vi "AMC100 UI.vi"() -> ()   [LabVIEW 2016]
panel:
  in  "stop":bool
  in  "Tab Control":enum32{"Navigation", "Interface", "About"}(tab)
  out "move out":bool caption="Move"
  in  "Positioner 2":u16(ring)=15 caption="Positioner" items=["ECGp5050", "ECGt5050", "ECR3030", "ECR4040", "ECR5050", "ECSx3030", "ECSx3040", "ECSx3050", "ECSx3060", "ECSx3070", "ECSx3080", "ECSx5050", "ECSxy5050", "ECSz3030", "ECSz5050", "EOP1", "EOP2"]
  out "in target range3":bool
  in  "Target Range 3":u32 caption="Target Range"
  in  "Reset Error 2":bool
  in  "Reset Error 3":bool
  out "Error 3":bool caption="Error"
  out "Error Message 3":string
  out "actor type 3":u16(ring) caption="Status" items=["linear positioner"=0, "goniometer"=1, "rotator"=2, "< error >"=9]
  out "actor type 2":u16(ring) caption="Status" items=["linear positioner"=0, "rotator"=1, "goniometer"=2, "< error >"=9]
  out "actor type":u16(ring) caption="Status" items=["linear positioner"=0, "rotator"=1, "goniometer"=2, "< error >"=9]
  out "EotLeftDetected3":bool caption="Status Eot BWD"
  out "EotrightDetected3":bool caption="Status Eot FWD"
  in  "EoT 3":bool=TRUE caption="Stop on EoT"
  out "EotLeftDetected2":bool caption="Status Eot BWD"
  out "EotrightDetected2":bool caption="Status Eot FWD"
  in  "EoT 2":bool=TRUE caption="Stop on EoT"
  in  "Move 3":bool
  out "MoveSignal 3":bool caption="Move"
  out "MoveSignal":bool caption="Move"
  out "ReferenceSignal":bool=TRUE
  in  "Axis 3":bool caption="Closed Loop Funktions"
  in  "Axis 2":bool caption="Closed Loop Funktions"
  in  "Target Position 3":i32 caption="Target Position [µm]"
  in  "Target Position 1":i32 caption="Target position [µm]"
  in  "Number of steps 3":i32=1 caption="Number of Steps"
  in  "Number of steps 2":i32=1 caption="Number of Steps"
  in  "Output 2":bool caption="Axis 2"
  in  "Move 2":bool
  in  "Move":bool
  out "ReferenceSignal 3":bool
  out "Reference 3":dbl caption="Reference position [µm]" format="%#_6f"
  in  "Output":bool=TRUE caption="Axis 1"
  out "Output Status 3":bool caption="Output Status"
  out "Error Message":string
  out "Error":bool
  in  "Output 3":bool caption="Axis 3"
  out "Output Status 1":bool=TRUE caption="Output Status"
  out "Position 3":dbl caption="Position [µm]" format="%#_10g"
  out "Output Status 2":bool caption="Output Status"
  in  "auto Reset 3":bool=TRUE caption="Auto Reset"
  in  "amplitude [V] 3":dbl=45.001 caption="Amplitude [V]" format="%#.3f"
  in  "frequency [Hz] 3":dbl=997.363 caption="Frequency [Hz]" format="%#.3f"
  out "Error 2":bool caption="Error"
  out "Error Message 2":string
  out "Connected 3":bool caption="Positioner Connected/Moving"
  in  "Single Step Left 3":bool caption="Open Loop Funktions"
  in  "Positioner 3":u16(ring)=15 caption="Positioner" items=["ECGp5050", "ECGt5050", "ECR3030", "ECR4040", "ECR5050", "ECSx3030", "ECSx3040", "ECSx3050", "ECSx3060", "ECSx3070", "ECSx3080", "ECSx5050", "ECSxy5050", "ECSz3030", "ECSz5050", "EOP1", "EOP2"]
  in  "Endless Left 3":bool caption="Continuous Backward"
  in  "Continuous Forward":bool
  in  "Single Step Right 3":bool caption="Step(s)"
  in  "Fixed DC 3":i32 caption="DC Level"
  out "move out 3":bool caption="Move"
  out "Position 2":i32 caption="Position [µm]"
  in  "amplitude [V] 2":dbl=45.001 caption="Amplitude [V]" format="%#.3f"
  in  "Reference Auto Update 3":bool=TRUE caption="Auto Update"
  in  "Amplitude [V]":dbl=45.001 format="%#.3f"
  in  "frequency [Hz] 2":dbl=997.363 caption="Frequency [Hz]" format="%#.3f"
  in  "Reference Auto Update 1":bool=TRUE caption="Auto Update"
  in  "Frequency [Hz]":dbl=1998.531 format="%#.3f"
  out "Connected 2":bool caption="Positioner Connected/Moving"
  in  "Single Step Left":bool caption="Open Loop Funktions"
  in  "Single Step Left 2":bool caption="Open Loop Funktions"
  in  "Single Step Right 2":bool caption="Step(s)"
  in  "Number of steps 1":i32=1 caption="Number of Steps"
  out "ReferenceSignal 2":bool
  in  "Single Step Right":bool caption="Step(s)"
  in  "Endless Left":bool caption="Continuous Backward"
  in  "Continuous Forward":bool
  in  "Endless Left 2":bool caption="Continuous Backward"
  out "EotLeftDetected1":bool caption="Status Eot BWD"
  out "EotrightDetected1":bool caption="Status Eot FWD"
  in  "EoT 1":bool caption="Stop on EoT"
  in  "Target position 2":i32 caption="Target Position [µm]"
  out "in target range2":bool
  in  "Continuous Forward":bool
  out "Reference 2":i32 caption="Reference position [µm]"
  in  "Fixed DC 2":i32 caption="DC Level"
  out "MoveSignal 2":bool caption="Move"
  out "in target range1":bool
  in  "Target Range 2":u32 caption="Target Range"
  in  "Target Range 1":u32 caption="Target Range"
  out "Reference":dbl=-7597148.0 caption="Reference position [µm]" format="%#_6f"
  out "Position":dbl=14701.126 caption="Position [µm]" format="%#_10f"
  in  "Axis 1":bool caption="Closed Loop Funktions"
  in  "auto Reset 1":bool=TRUE caption="Auto Reset"
  in  "Fixed DC 1":i32 caption="DC Level"
  out "move out 2":bool caption="Move"
  in  "auto Reset 2":bool=TRUE caption="Auto Reset"
  in  "Reference Auto Update 2":bool=TRUE caption="Auto Update"
  in  "Reset Error":bool
  out "Connected":bool=TRUE caption="Positioner Connected/Moving"
  in  "Positioner":u16(ring)=15 items=["ECGp5050", "ECGt5050", "ECR3030", "ECR4040", "ECR5050", "ECSx3030", "ECSx3040", "ECSx3050", "ECSx3060", "ECSx3070", "ECSx3080", "ECSx5050", "ECSxy5050", "ECSz3030", "ECSz5050", "EOP1", "EOP2"]
  in  "RT in move 3":bool=TRUE caption="Move"
  in  "Steps per pulse 3":i32 caption="Steps per pulse [Steps]"
  out "RT in move Signal 3":bool=TRUE caption="move"
  in  "Mode Input 3":u16(ring) caption="Mode" items=["Trigger (LVDS)"=11, "Trigger (LVTTL)"=10, "Stepper (LVDS)"=9, "Stepper (LVTTL)"=8, "AquadB (LVDS)"=1, "AquadB (LVTTL)"=0, "OFF"=15]
  in  "Loop Mode 3":u16(ring) caption="Loop mode" items=["closed-loop"=1, "open-loop"=0]
  in  "Change per pulse 3":i32 caption="Change per pulse  [u°/nm]"
  in  "RT in move 2":bool=TRUE caption="Move"
  in  "Steps per pulse 2":i32 caption="Steps per pulse [Steps]"
  out "RT in move Signal 2":bool=TRUE caption="move"
  in  "Mode Input 2":u16(ring) caption="Mode" items=["Trigger (LVDS)"=11, "Trigger (LVTTL)"=10, "Stepper (LVDS)"=9, "Stepper (LVTTL)"=8, "AquadB (LVDS)"=1, "AquadB (LVTTL)"=0, "OFF"=15]
  in  "Loop Mode 2":u16(ring) caption="Loop mode" items=["closed-loop"=1, "open-loop"=0]
  in  "Change per pulse 2":i32 caption="Change per pulse  [u°/nm]"
  in  "Output Mode":u16(ring) caption="Mode" items=["AquadB (LVTTL)", "AquadB (LVDS)"]
  in  "RT in move 1":bool=TRUE caption="Move"
  in  "AquadB Resolution 3":i32 caption="AquadB Resolution [nm]"
  in  "AqaudB clock 2":i32 caption="AquadB Clock [ns]"
  in  "AqaudB clock 1":i32 caption="AquadB Clock [ns]"
  in  "AquadB Resolution 2":i32 caption="AquadB Resolution [nm]"
  in  "AquadB out 1":bool caption="AquadB enable"
  in  "Steps per pulse 1":i32 caption="Steps per pulse [Steps]"
  in  "AquadB out 3":bool caption="AquadB enable"
  in  "AquadB in res 1":i32 caption="AquadB Resolution [nm]"
  in  "AquadB Resolution 1":i32 caption="AquadB Resolution [nm]"
  in  "AquadB out 2":bool caption="AquadB enable"
  in  "AqaudB clock 3":i32 caption="AquadB Clock [ns]"
  in  "Reset Error 6":bool
  in  "Reset Error 5":bool
  out "Error Message 5":string
  out "Error 5":bool caption="Error"
  out "Error Message 6":string
  out "Error 6":bool caption="Error"
  in  "AquadB in res 3":i32 caption="AquadB Resolution [nm]"
  in  "AquadB in res 2":i32 caption="AquadB Resolution [nm]"
  in  "Reset Error 4":bool
  out "RT in move Signal 1":bool=TRUE caption="move"
  in  "Mode Input 1":u16(ring) caption="Mode" items=["Trigger (LVDS)"=11, "Trigger (LVTTL)"=10, "Stepper (LVDS)"=9, "Stepper (LVTTL)"=8, "AquadB (LVDS)"=1, "AquadB (LVTTL)"=0, "OFF"=15]
  out "Error Message 4":string
  out "Error 4":bool caption="Error"
  in  "Loop Mode 1":u16(ring) caption="Loop mode" items=["closed-loop"=1, "open-loop"=0]
  in  "Change per pulse 1":i32 caption="Change per pulse [u°/nm]"
  in  "Reset Error 7":bool
  in  "Factory Reset":bool
  in  "Reboot":bool
  out "Error Message 7":string
  in  "Lock password":string
  in  "name":string caption="Device Name"
  in  "Access Password":string
  out "locked":bool
  out "authorized":bool
  out "Error 7":bool caption="Error"
  in  "Unlock":bool=TRUE
  out "Name":string caption="Device Name"
  out "Device type":string="AMC100/NUM"
  out "Mac Adress":string="70:B3:D5:D7:61:E1"
  out "Sn":string caption="Serial Number"
  out "ip":string="192.168.1.1" caption="IP Adress"
  out "Firmware":string caption="Firmware Version"
  out "FPGA":string caption="FPGA Version"
  # "Real Time Output"
  # "Real Time Input"
  # "Global Parameters"
  # "Axis 1"
  # "Axis 1"
  # "Axis 2"
  # "Axis 2"
  # "Axis 3"
  # "Axis 3"
  # "Device Info"
  # "Device Access"
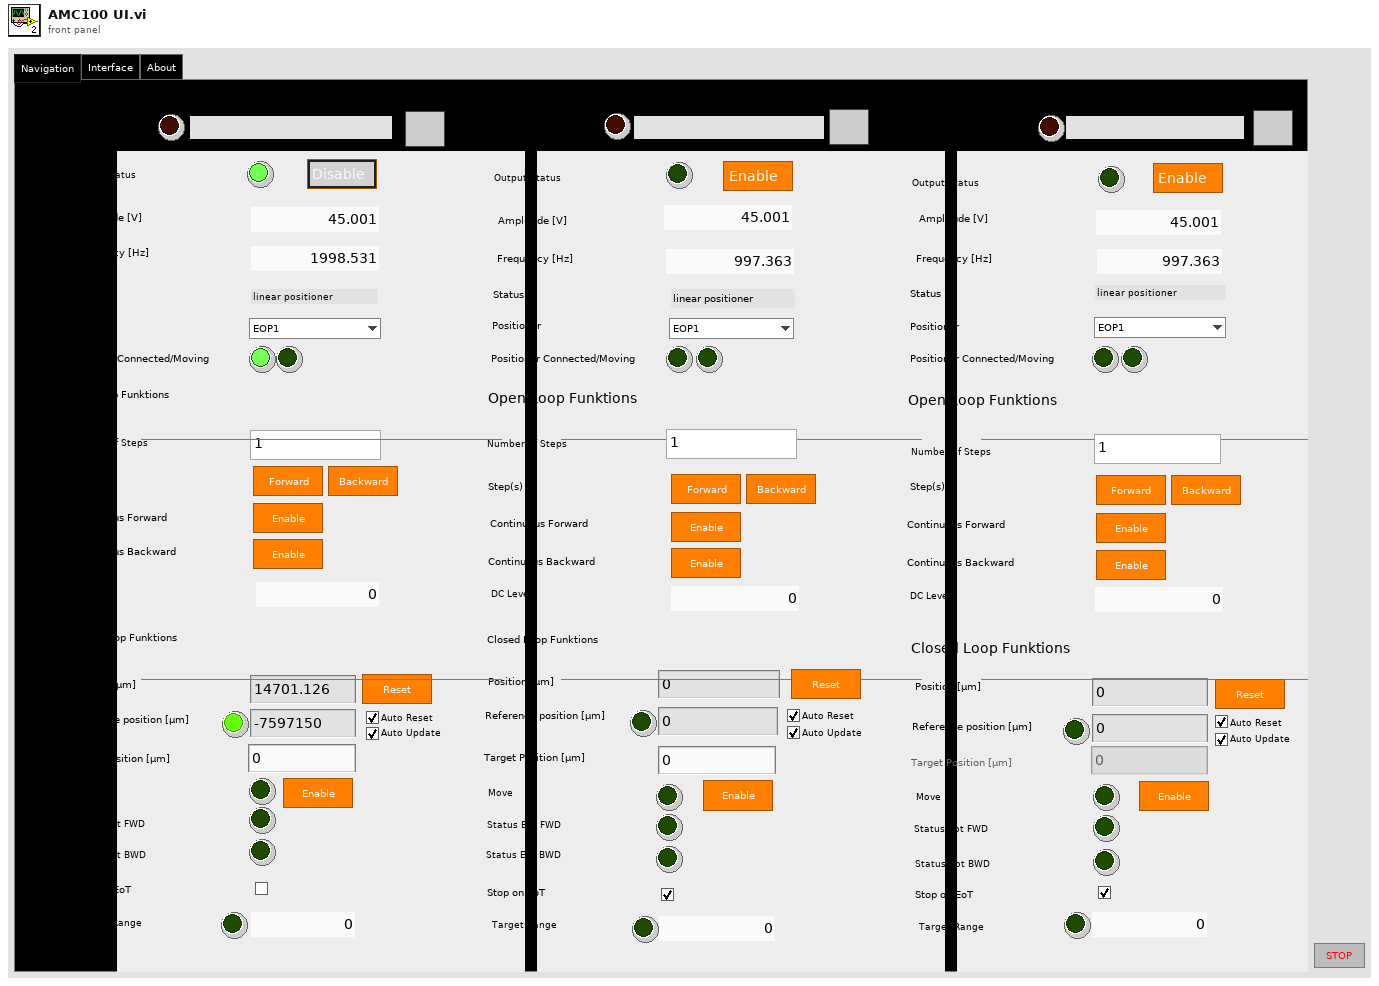
[diagram p1: front panel]
types:
  T1 = enum8{"Enabled", "Disabled", "Disabled and Grayed Out"}
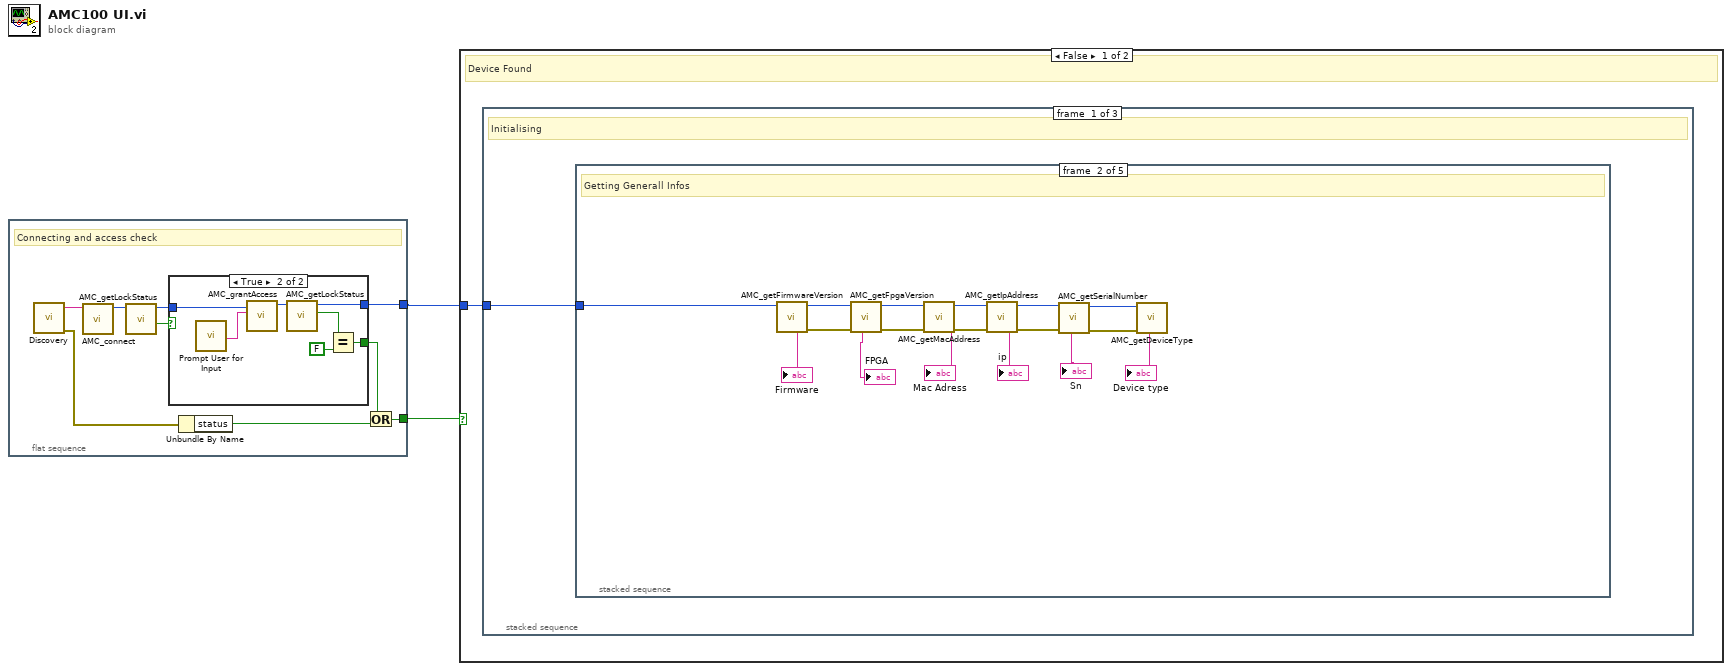
[diagram p0: block diagram]
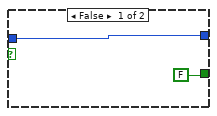
[diagram p2: hidden frame]
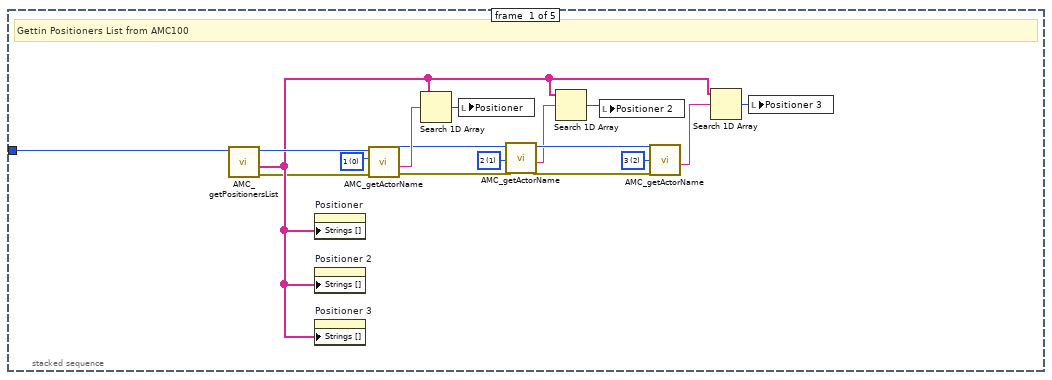
[diagram p3: hidden frame]
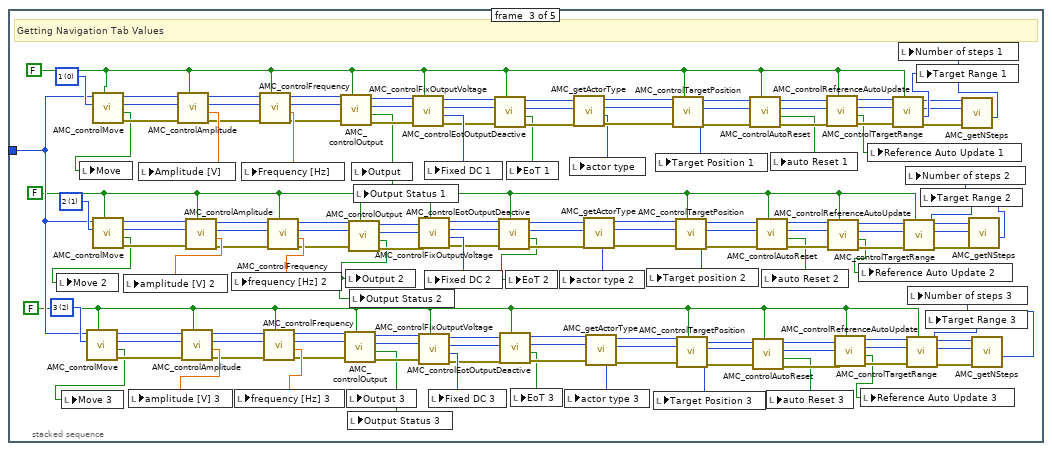
[diagram p4: hidden frame]
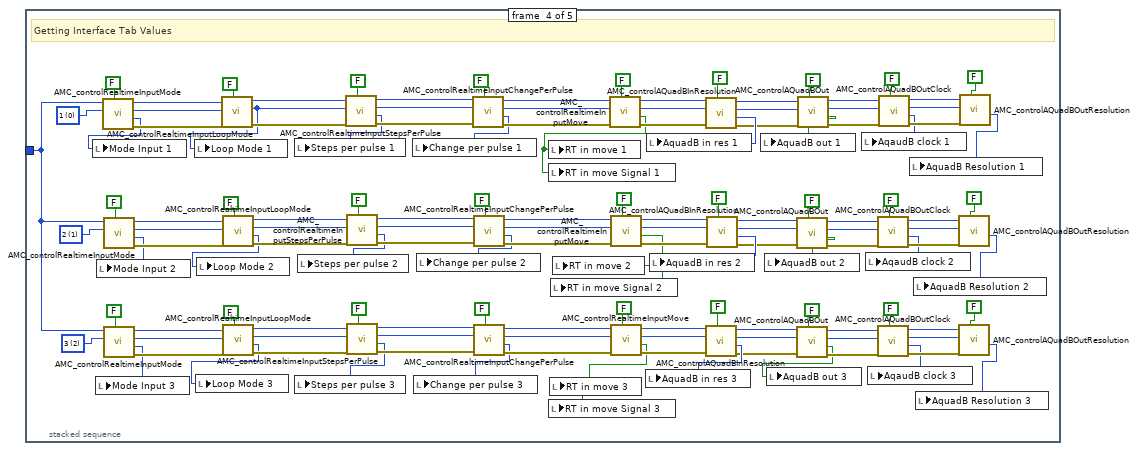
[diagram p5: hidden frame]
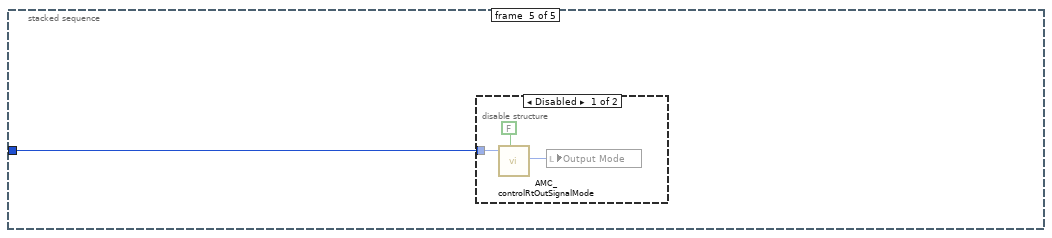
[diagram p6: hidden frame]
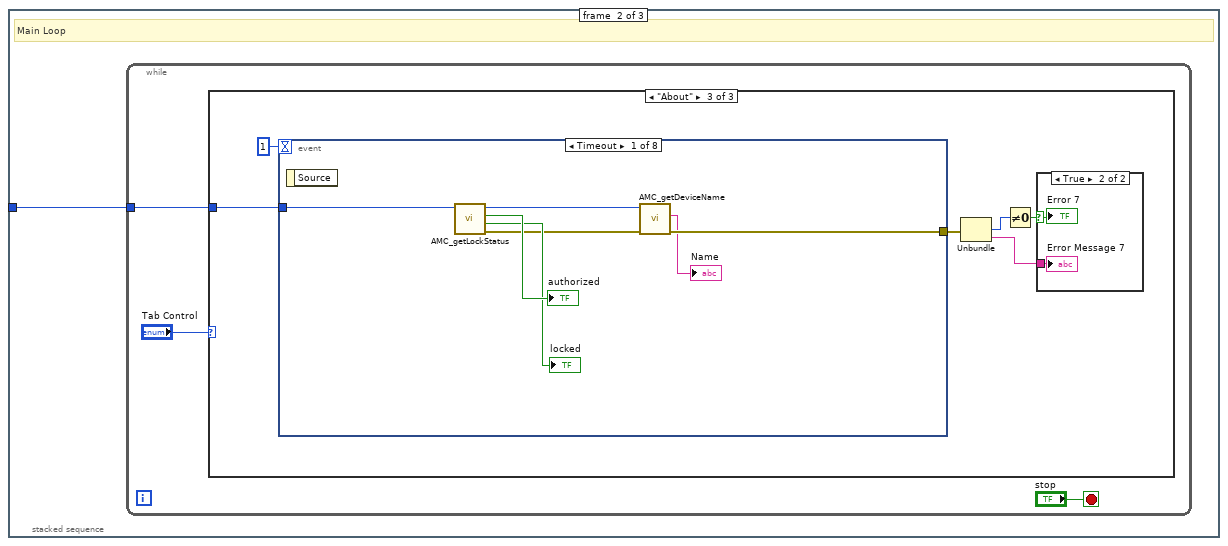
[diagram p8: hidden frame]
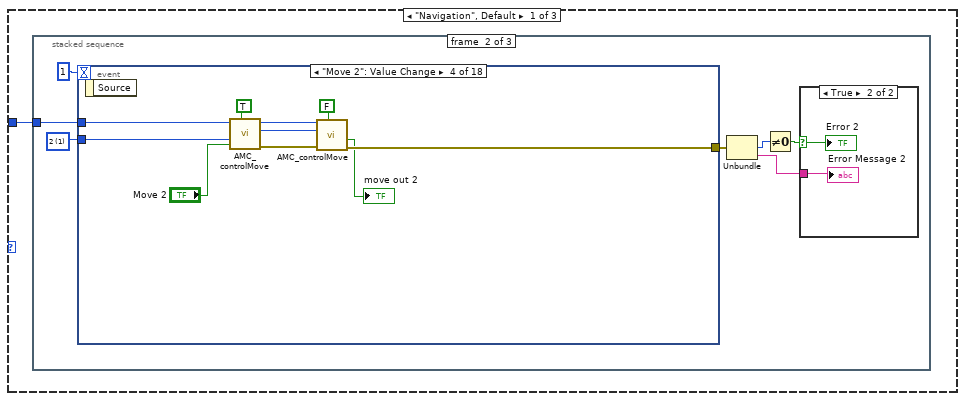
[diagram p9: hidden frame]
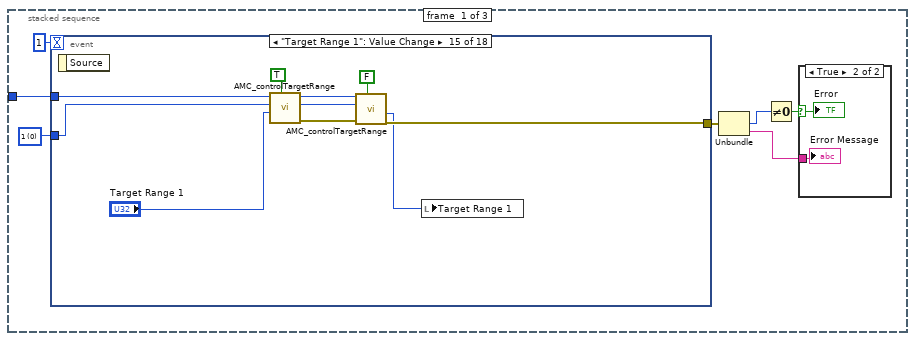
[diagram p10: hidden frame]
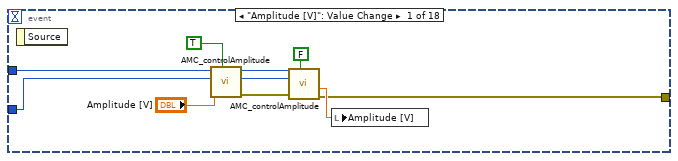
[diagram p12: hidden frame]
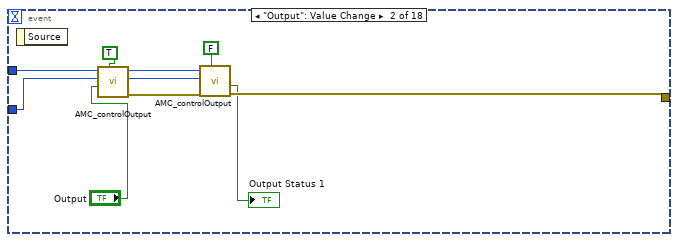
[diagram p13: hidden frame]
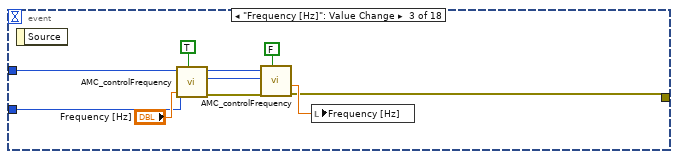
[diagram p14: hidden frame]
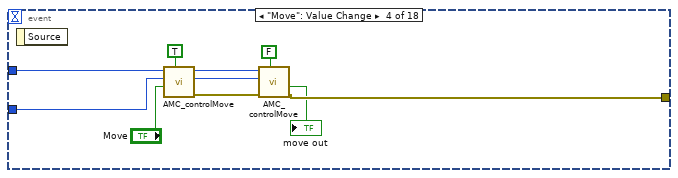
[diagram p15: hidden frame]
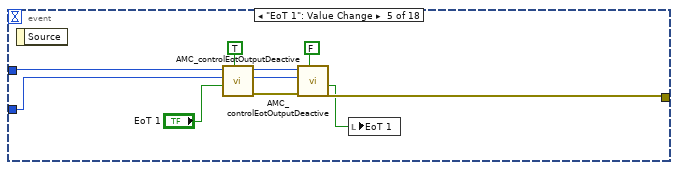
[diagram p16: hidden frame]
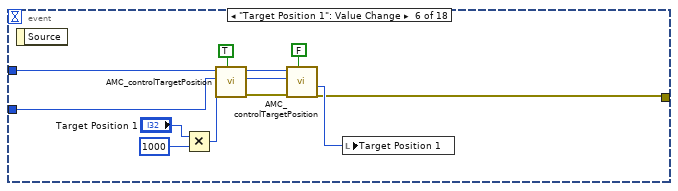
[diagram p17: hidden frame]
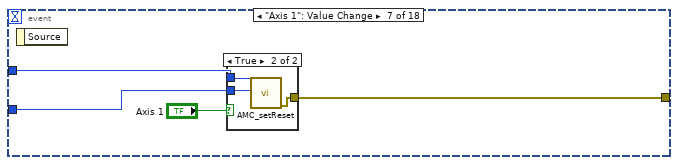
[diagram p18: hidden frame]
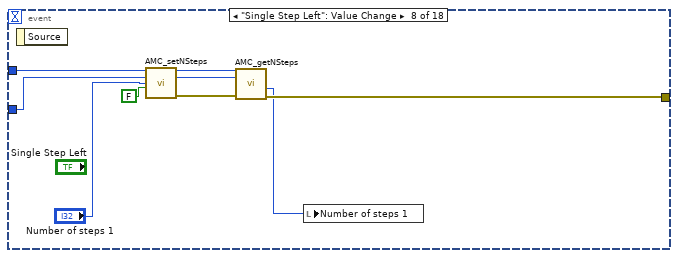
[diagram p20: hidden frame]
diagram:
  n1 = flat-sequence {
    tunnel: [w10] -> w1
    tunnel: [w11] -> w2
    frame #0 {
      # "Connecting and access check"
      n2 = call "Discovery.vi"() -> ("error out"=w3:errorcluster, "IP"=w4:string)  [unwired: 10 in]
      n3 = call "AMC_connect.vi"("deviceAddress"=w4) -> ("deviceHandle"=w7:i32)  [unwired: 5 in, 1 out]
      n4 = call "AMC_getLockStatus.vi"("deviceHandle"=w7) -> ("locked"=w5:bool, "deviceHandle"=w6:i32)  [unwired: 7 in, 2 out]
      n5 = case shown="True" w5 {
        tunnel: w6 -> [w13 w20]
        tunnel: [w13 w17] -> w11
        tunnel: [FALSE w14] -> w9
        frame False {
        }
        frame True {
          n6 = call "Prompt User for Input"() -> ("password"=w19:string)  [unwired: 17 in, 2 out]
          n7 = call "AMC_grantAccess.vi"("password"=w19, "deviceHandle"=w20) -> ("deviceHandle"=w18:i32)  [unwired: 8 in, 1 out]
          n8 = call "AMC_getLockStatus.vi"("deviceHandle"=w18) -> ("authorized"=w15:bool, "deviceHandle"=w17:i32)  [unwired: 7 in, 2 out]
          n9 = Equal?(x=w15, y=FALSE) -> (x = y?=w14:bool)
        }
      }
      n10 = Unbundle By Name(w3) -> ("status"=w8:bool)
      n11 = Or(x=w9, y=w8) -> (x .or. y?=w10:bool)
    }
  }
  n12 = case shown="False" w1 {
    tunnel: w2 -> [w21 _]
    frame False {
      # "Device Found"
      n13 = stacked-sequence {
        tunnel: w21 -> [w22 w332 w1333]
        frame #0 {
          # "Initialising"
          n14 = stacked-sequence {
            tunnel: w22 -> [w32 w44 w102 w278 w328]
            frame #0 {
              w34 = u8 2 items=["1", "2", "3"] ("axis")
              w33 = u8 1 items=["1", "2", "3"] ("axis")
              w37 = u8 0 items=["1", "2", "3"] ("axis")
              # "Gettin Positioners List from AMC100"
              n15 = call "AMC_getPositionersList.vi"("deviceHandle"=w32) -> ("error out"=w23:errorcluster, "list"=w26:string[], "deviceHandle"=w27:i32)  [unwired: 7 in, 1 out]
              n16 = property on="Positioner" class="Ring (strict)"("Strings []"=w26) -> ()  [unwired: 2 in, 2 out]
              n17 = property on="Positioner 2" class="Ring (strict)"("Strings []"=w26) -> ()  [unwired: 2 in, 2 out]
              n18 = property on="Positioner 3" class="Ring (strict)"("Strings []"=w26) -> ()  [unwired: 2 in, 2 out]
              n19 = call "AMC_getActorName.vi"("error in"=w23, "axis"=w37, "deviceHandle"=w27) -> ("error out"=w25:errorcluster, "actor name"=w38:string, "deviceHandle"=w36:i32)  [unwired: 5 in, 1 out]
              n20 = Search 1D Array(1D array=w26, element=w38) -> (index of element=w39:i32)  [unwired: 1 in]
              n21 = local write "Positioner"(w39) -> ()
              n22 = call "AMC_getActorName.vi"("error in"=w25, "axis"=w33, "deviceHandle"=w36) -> ("error out"=w24:errorcluster, "actor name"=w29:string, "deviceHandle"=w35:i32)  [unwired: 5 in, 1 out]
              n23 = Search 1D Array(1D array=w26, element=w29) -> (index of element=w31:i32)  [unwired: 1 in]
              n24 = local write "Positioner 2"(w31) -> ()
              n25 = call "AMC_getActorName.vi"("error in"=w24, "axis"=w34, "deviceHandle"=w35) -> ("actor name"=w28:string)  [unwired: 5 in, 3 out]
              n26 = Search 1D Array(1D array=w26, element=w28) -> (index of element=w30:i32)  [unwired: 1 in]
              n27 = local write "Positioner 3"(w30) -> ()
            }
            frame #1 {
              # "Getting Generall Infos"
              n28 = call "AMC_getFirmwareVersion.vi"("deviceHandle"=w44) -> ("error out"=w42:errorcluster, "version"=→"Firmware":string, "deviceHandle"=w43:i32)  [unwired: 8 in]
              n29 = call "AMC_getFpgaVersion.vi"("error in"=w42, "device Handle"=w43) -> ("error out"=w52:errorcluster, "version"=→"FPGA":string, "device Handle"=w56:i32)  [unwired: 7 in]
              n30 = call "AMC_getMacAddress.vi"("error in"=w52, "deviceHandle"=w56) -> ("error out"=w51:errorcluster, "mac"=→"Mac Adress":string, "deviceHandle"=w54:i32)  [unwired: 7 in]
              n31 = call "AMC_getIpAddress.vi"("error in"=w51, "device Handle"=w54) -> ("error out"=w48:errorcluster, "ip"=→"ip":string, "device Handle"=w49:i32)  [unwired: 7 in]
              n32 = call "AMC_getSerialNumber.vi"("error in"=w48, "device Handle"=w49) -> ("error out"=w45:errorcluster, "sn"=→"Sn":string, "device Handle"=w46:i32)  [unwired: 7 in]
              n33 = call "AMC_getDeviceType.vi"("error in"=w45, "device Handle"=w46) -> ("type"=→"Device type":string)  [unwired: 7 in, 2 out]
            }
            frame #2 {
              w103 = u8 2 items=["1", "2", "3"] ("axis")
              w90 = FALSE ("set")
              w104 = u8 1 items=["1", "2", "3"] ("axis")
              w91 = FALSE ("set")
              w105 = u8 0 items=["1", "2", "3"] ("axis")
              w92 = FALSE ("set")
              # "Getting Navigation Tab Values"
              n34 = call "AMC_controlMove.vi"("set"=w90, "axis"=w103, "deviceHandle"=w102) -> ("error out"=w106:errorcluster, "enable out"=w73:bool, "axis"=w107:u8, "deviceHandle"=w108:i32)  [unwired: 5 in]
              n35 = local write "Move 3"(w73) -> ()
              n36 = call "AMC_controlMove.vi"("set"=w92, "axis"=w105, "deviceHandle"=w102) -> ("error out"=w114:errorcluster, "enable out"=w83:bool, "axis"=w112:u8, "deviceHandle"=w113:i32)  [unwired: 5 in]
              n37 = local write "Move"(w83) -> ()
              n38 = call "AMC_controlMove.vi"("set"=w91, "axis"=w104, "deviceHandle"=w102) -> ("error out"=w109:errorcluster, "enable out"=w78:bool, "axis"=w110:u8, "deviceHandle"=w111:i32)  [unwired: 5 in]
              n39 = local write "Move 2"(w78) -> ()
              n40 = call "AMC_controlAmplitude.vi"("set"=w92, "error in"=w114, "axis"=w112, "deviceHandle"=w113) -> ("error out"=w171:errorcluster, "amplitude [V] out"=w197:dbl, "axis"=w183:u8, "deviceHandle"=w198:i32)  [unwired: 2 in]
              n41 = local write "Amplitude [V]"(w197) -> ()
              n42 = call "AMC_controlAmplitude.vi"("set"=w90, "error in"=w106, "axis"=w107, "deviceHandle"=w108) -> ("error out"=w165:errorcluster, "amplitude [V] out"=w188:dbl, "axis"=w177:u8, "deviceHandle"=w192:i32)  [unwired: 2 in]
              n43 = local write "amplitude [V] 3"(w188) -> ()
              n44 = call "AMC_controlAmplitude.vi"("set"=w91, "error in"=w109, "axis"=w110, "deviceHandle"=w111) -> ("error out"=w168:errorcluster, "amplitude [V] out"=w190:dbl, "axis"=w180:u8, "deviceHandle"=w194:i32)  [unwired: 2 in]
              n45 = local write "amplitude [V] 2"(w190) -> ()
              n46 = call "AMC_controlFrequency.vi"("set"=w92, "error in"=w171, "axis"=w183, "deviceHandle"=w198) -> ("error out"=w170:errorcluster, "frequency [Hz] out"=w196:dbl, "axis"=w182:u8, "deviceHandle"=w195:i32)  [unwired: 4 in]
              n47 = local write "Frequency [Hz]"(w196) -> ()
              n48 = call "AMC_controlFrequency.vi"("set"=w90, "error in"=w165, "axis"=w177, "deviceHandle"=w192) -> ("error out"=w164:errorcluster, "frequency [Hz] out"=w187:dbl, "axis"=w176:u8, "deviceHandle"=w191:i32)  [unwired: 4 in]
              n49 = local write "frequency [Hz] 3"(w187) -> ()
              n50 = call "AMC_controlFrequency.vi"("set"=w91, "error in"=w168, "axis"=w180, "deviceHandle"=w194) -> ("error out"=w167:errorcluster, "frequency [Hz] out"=w189:dbl, "axis"=w179:u8, "deviceHandle"=w193:i32)  [unwired: 4 in]
              n51 = local write "frequency [Hz] 2"(w189) -> ()
              n52 = call "AMC_controlOutput.vi"("set"=w92, "error in"=w170, "axis"=w182, "deviceHandle"=w195) -> ("error out"=w169:errorcluster, "enable out"=w82:bool, "axis"=w181:u8, "deviceHandle"=w186:i32)  [unwired: 4 in]
              n53 = call "AMC_controlOutput.vi"("set"=w90, "error in"=w164, "axis"=w176, "deviceHandle"=w191) -> ("error out"=w163:errorcluster, "enable out"=w72:bool, "axis"=w175:u8, "deviceHandle"=w184:i32)  [unwired: 4 in]
              n54 = local write "Output 3"(w72) -> ()
              n55 = local write "Output Status 3"(w72) -> ()
              n56 = call "AMC_controlOutput.vi"("set"=w91, "error in"=w167, "axis"=w179, "deviceHandle"=w193) -> ("error out"=w166:errorcluster, "enable out"=w77:bool, "axis"=w178:u8, "deviceHandle"=w185:i32)  [unwired: 4 in]
              n57 = local write "Output 2"(w77) -> ()
              n58 = local write "Output Status 2"(w77) -> ()
              n59 = local write "Output"(w82) -> ()
              n60 = local write "Output Status 1"(w82) -> ()
              n61 = call "AMC_controlFixOutputVoltage.vi"("set"=w92, "error in"=w169, "axis"=w181, "deviceHandle"=w186) -> ("error out"=w160:errorcluster, "voltage"=w174:i32, "axis"=w161:u8, "deviceHandle"=w162:i32)  [unwired: 4 in]
              n62 = call "AMC_controlFixOutputVoltage.vi"("set"=w91, "error in"=w166, "axis"=w178, "deviceHandle"=w185) -> ("error out"=w157:errorcluster, "voltage"=w173:i32, "axis"=w158:u8, "deviceHandle"=w159:i32)  [unwired: 4 in]
              n63 = call "AMC_controlFixOutputVoltage.vi"("set"=w90, "error in"=w163, "axis"=w175, "deviceHandle"=w184) -> ("error out"=w154:errorcluster, "voltage"=w172:i32, "axis"=w155:u8, "deviceHandle"=w156:i32)  [unwired: 4 in]
              n64 = local write "Fixed DC 1"(w174) -> ()
              n65 = local write "Fixed DC 2"(w173) -> ()
              n66 = local write "Fixed DC 3"(w172) -> ()
              n67 = call "AMC_controlEotOutputDeactive.vi"("set"=w92, "error in"=w160, "axis"=w161, "deviceHandle"=w162) -> ("error out"=w151:errorcluster, "enable out"=w81:bool, "axis"=w152:u8, "deviceHandle"=w153:i32)  [unwired: 4 in]
              n68 = call "AMC_controlEotOutputDeactive.vi"("set"=w91, "error in"=w157, "axis"=w158, "deviceHandle"=w159) -> ("error out"=w148:errorcluster, "enable out"=w76:bool, "axis"=w149:u8, "deviceHandle"=w150:i32)  [unwired: 4 in]
              n69 = call "AMC_controlEotOutputDeactive.vi"("set"=w90, "error in"=w154, "axis"=w155, "deviceHandle"=w156) -> ("error out"=w145:errorcluster, "enable out"=w71:bool, "axis"=w146:u8, "deviceHandle"=w147:i32)  [unwired: 4 in]
              n70 = local write "EoT 2"(w76) -> ()
              n71 = local write "EoT 1"(w81) -> ()
              n72 = local write "EoT 3"(w71) -> ()
              n73 = call "AMC_getActorType.vi"("error in"=w151, "axis"=w152, "deviceHandle"=w153) -> ("error out"=w139:errorcluster, "positioner type"=w86:u16, "axis"=w140:i32, "deviceHandle"=w141:i32)  [unwired: 5 in]
              n74 = local write "actor type"(w86) -> ()
              n75 = call "AMC_getActorType.vi"("error in"=w148, "axis"=w149, "deviceHandle"=w150) -> ("error out"=w142:errorcluster, "positioner type"=w85:u16, "axis"=w143:i32, "deviceHandle"=w144:i32)  [unwired: 5 in]
              n76 = local write "actor type 2"(w85) -> ()
              n77 = call "AMC_getActorType.vi"("error in"=w145, "axis"=w146, "deviceHandle"=w147) -> ("error out"=w136:errorcluster, "positioner type"=w84:u16, "axis"=w137:i32, "deviceHandle"=w138:i32)  [unwired: 5 in]
              n78 = local write "actor type 3"(w84) -> ()
              n79 = call "AMC_controlTargetPosition.vi"("set"=w92, "error in"=w139, "axis"=w140, "deviceHandle"=w141) -> ("error out"=w132:errorcluster, "target out"=w135:i32, "axis"=w128:u8, "deviceHandle"=w130:i32)  [unwired: 4 in]
              n80 = local write "Target Position 1"(w135) -> ()
              n81 = call "AMC_controlTargetPosition.vi"("set"=w91, "error in"=w142, "axis"=w143, "deviceHandle"=w144) -> ("error out"=w126:errorcluster, "target out"=w134:i32, "axis"=w122:u8, "deviceHandle"=w124:i32)  [unwired: 4 in]
              n82 = local write "Target position 2"(w134) -> ()
              n83 = call "AMC_controlTargetPosition.vi"("set"=w90, "error in"=w136, "axis"=w137, "deviceHandle"=w138) -> ("error out"=w120:errorcluster, "target out"=w133:i32, "axis"=w116:u8, "deviceHandle"=w118:i32)  [unwired: 4 in]
              n84 = local write "Target Position 3"(w133) -> ()
              n85 = call "AMC_controlAutoReset.vi"("set"=w92, "error in"=w132, "axis"=w128, "deviceHandle in"=w130) -> ("error out"=w131:errorcluster, "enable out"=w80:bool, "axis"=w127:u8, "deviceHandle out"=w129:i32)  [unwired: 4 in]
              n86 = call "AMC_controlAutoReset.vi"("set"=w90, "error in"=w120, "axis"=w116, "deviceHandle in"=w118) -> ("error out"=w119:errorcluster, "enable out"=w70:bool, "axis"=w115:u8, "deviceHandle out"=w117:i32)  [unwired: 4 in]
              n87 = call "AMC_controlAutoReset.vi"("set"=w91, "error in"=w126, "axis"=w122, "deviceHandle in"=w124) -> ("error out"=w125:errorcluster, "enable out"=w75:bool, "axis"=w121:u8, "deviceHandle out"=w123:i32)  [unwired: 4 in]
              n88 = local write "auto Reset 2"(w75) -> ()
              n89 = local write "auto Reset 3"(w70) -> ()
              n90 = local write "auto Reset 1"(w80) -> ()
              n91 = call "AMC_controlReferenceAutoUpdate.vi"("set"=w92, "error in"=w131, "axis"=w127, "deviceHandle"=w129) -> ("error out"=w99:errorcluster, "enable out"=w79:bool, "axis"=w100:u8, "deviceHandle"=w101:i32)  [unwired: 4 in]
              n92 = call "AMC_controlReferenceAutoUpdate.vi"("set"=w91, "error in"=w125, "axis"=w121, "deviceHandle"=w123) -> ("error out"=w96:errorcluster, "enable out"=w74:bool, "axis"=w97:u8, "deviceHandle"=w98:i32)  [unwired: 4 in]
              n93 = call "AMC_controlReferenceAutoUpdate.vi"("set"=w90, "error in"=w119, "axis"=w115, "deviceHandle"=w117) -> ("error out"=w93:errorcluster, "enable out"=w69:bool, "axis"=w94:u8, "deviceHandle"=w95:i32)  [unwired: 4 in]
              n94 = local write "Reference Auto Update 2"(w74) -> ()
              n95 = local write "Reference Auto Update 3"(w69) -> ()
              n96 = local write "Reference Auto Update 1"(w79) -> ()
              n97 = call "AMC_controlTargetRange.vi"("set"=w92, "error in"=w99, "axis"=w100, "deviceHandle"=w101) -> ("error out"=w66:errorcluster, "range out"=w89:u32, "axis"=w67:u8, "deviceHandle"=w68:i32)  [unwired: 4 in]
              n98 = call "AMC_controlTargetRange.vi"("set"=w91, "error in"=w96, "axis"=w97, "deviceHandle"=w98) -> ("error out"=w58:errorcluster, "range out"=w88:u32, "axis"=w64:u8, "deviceHandle"=w65:i32)  [unwired: 4 in]
              n99 = call "AMC_controlTargetRange.vi"("set"=w90, "error in"=w93, "axis"=w94, "deviceHandle"=w95) -> ("error out"=w57:errorcluster, "range out"=w87:u32, "axis"=w62:u8, "deviceHandle"=w63:i32)  [unwired: 4 in]
              n100 = local write "Target Range 1"(w89) -> ()
              n101 = local write "Target Range 2"(w88) -> ()
              n102 = local write "Target Range 3"(w87) -> ()
              n103 = call "AMC_getNSteps.vi"("error in"=w66, "axis"=w67, "deviceHandle"=w68) -> ("n out"=w60:i32)  [unwired: 5 in, 3 out]
              n104 = local write "Number of steps 1"(w60) -> ()
              n105 = call "AMC_getNSteps.vi"("error in"=w58, "axis"=w64, "deviceHandle"=w65) -> ("n out"=w61:i32)  [unwired: 5 in, 3 out]
              n106 = local write "Number of steps 2"(w61) -> ()
              n107 = call "AMC_getNSteps.vi"("error in"=w57, "axis"=w62, "deviceHandle"=w63) -> ("n out"=w59:i32)  [unwired: 5 in, 3 out]
              n108 = local write "Number of steps 3"(w59) -> ()
            }
            frame #3 {
              w276 = u8 2 items=["1", "2", "3"] ("axis")
              w277 = u8 1 items=["1", "2", "3"] ("axis")
              w311 = u8 0 items=["1", "2", "3"] ("axis")
              # "Getting Interface Tab Values"
              n109 = call "AMC_controlRealtimeInputMode.vi"("set"=FALSE, "axis"=w311, "deviceHandle"=w278) -> ("error out"=w316:errorcluster, "mode out"=w261:i32, "axis"=w275:u8, "deviceHandle"=w321:i32)  [unwired: 5 in]
              n110 = local write "Mode Input 1"(w261) -> ()
              n111 = call "AMC_controlRealtimeInputMode.vi"("set"=FALSE, "axis"=w277, "deviceHandle"=w278) -> ("error out"=w306:errorcluster, "mode out"=w255:i32, "axis"=w271:u8, "deviceHandle"=w301:i32)  [unwired: 5 in]
              n112 = local write "Mode Input 2"(w255) -> ()
              n113 = call "AMC_controlRealtimeInputMode.vi"("set"=FALSE, "axis"=w276, "deviceHandle"=w278) -> ("error out"=w283:errorcluster, "mode out"=w249:i32, "axis"=w266:u8, "deviceHandle"=w288:i32)  [unwired: 5 in]
              n114 = local write "Mode Input 3"(w249) -> ()
              n115 = call "AMC_controlRealtimeInputLoopMode.vi"("set"=FALSE, "error in"=w316, "axis"=w275, "deviceHandle"=w321) -> ("error out"=w315:errorcluster, "axis"=w260:u8, "deviceHandle"=w320:i32)  [unwired: 4 in, 1 out]
              n116 = local write "Loop Mode 1"(w260) -> ()
              n117 = call "AMC_controlRealtimeInputLoopMode.vi"("set"=FALSE, "error in"=w306, "axis"=w271, "deviceHandle"=w301) -> ("error out"=w307:errorcluster, "mode out"=w254:i32, "axis"=w270:u8, "deviceHandle"=w302:i32)  [unwired: 4 in]
              n118 = local write "Loop Mode 2"(w254) -> ()
              n119 = call "AMC_controlRealtimeInputLoopMode.vi"("set"=FALSE, "error in"=w283, "axis"=w266, "deviceHandle"=w288) -> ("error out"=w282:errorcluster, "mode out"=w248:i32, "axis"=w265:u8, "deviceHandle"=w287:i32)  [unwired: 4 in]
              n120 = local write "Loop Mode 3"(w248) -> ()
              n121 = call "AMC_controlRealtimeInputStepsPerPulse.vi"("set"=FALSE, "error in"=w315, "axis"=w260, "deviceHandle"=w320) -> ("error out"=w314:errorcluster, "steps out"=w259:i32, "axis"=w274:u8, "deviceHandle"=w319:i32)  [unwired: 4 in]
              n122 = local write "Steps per pulse 1"(w259) -> ()
              n123 = call "AMC_controlRealtimeInputStepsPerPulse.vi"("set"=FALSE, "error in"=w307, "axis"=w270, "deviceHandle"=w302) -> ("error out"=w308:errorcluster, "steps out"=w253:i32, "axis"=w269:u8, "deviceHandle"=w303:i32)  [unwired: 4 in]
              n124 = local write "Steps per pulse 2"(w253) -> ()
              n125 = call "AMC_controlRealtimeInputStepsPerPulse.vi"("set"=FALSE, "error in"=w282, "axis"=w265, "deviceHandle"=w287) -> ("error out"=w281:errorcluster, "steps out"=w247:i32, "axis"=w264:u8, "deviceHandle"=w286:i32)  [unwired: 4 in]
              n126 = local write "Steps per pulse 3"(w247) -> ()
              n127 = call "AMC_controlRealtimeInputChangePerPulse.vi"("set"=FALSE, "error in"=w314, "axis"=w274, "deviceHandle"=w319) -> ("error out"=w313:errorcluster, "change out"=w258:i32, "axis"=w273:u8, "deviceHandle"=w318:i32)  [unwired: 4 in]
              n128 = local write "Change per pulse 1"(w258) -> ()
              n129 = call "AMC_controlRealtimeInputChangePerPulse.vi"("set"=FALSE, "error in"=w308, "axis"=w269, "deviceHandle"=w303) -> ("error out"=w309:errorcluster, "change out"=w252:i32, "axis"=w268:u8, "deviceHandle"=w304:i32)  [unwired: 4 in]
              n130 = local write "Change per pulse 2"(w252) -> ()
              n131 = call "AMC_controlRealtimeInputChangePerPulse.vi"("set"=FALSE, "error in"=w281, "axis"=w264, "deviceHandle"=w286) -> ("error out"=w280:errorcluster, "change out"=w246:i32, "axis"=w263:u8, "deviceHandle"=w285:i32)  [unwired: 4 in]
              n132 = local write "Change per pulse 3"(w246) -> ()
              n133 = call "AMC_controlRealtimeInputMove.vi"("set"=FALSE, "error in"=w313, "axis"=w273, "deviceHandle"=w318) -> ("error out"=w312:errorcluster, "enable out"=w257:bool, "axis"=w272:u8, "deviceHandle"=w317:i32)  [unwired: 4 in]
              n134 = local write "RT in move 1"(w257) -> ()
              n135 = local write "RT in move Signal 1"(w257) -> ()
              n136 = call "AMC_controlRealtimeInputMove.vi"("set"=FALSE, "error in"=w309, "axis"=w268, "deviceHandle"=w304) -> ("error out"=w310:errorcluster, "enable out"=w251:bool, "axis"=w267:u8, "deviceHandle"=w305:i32)  [unwired: 4 in]
              n137 = local write "RT in move Signal 2"(w251) -> ()
              n138 = local write "RT in move 2"(w251) -> ()
              n139 = call "AMC_controlRealtimeInputMove.vi"("set"=FALSE, "error in"=w280, "axis"=w263, "deviceHandle"=w285) -> ("error out"=w279:errorcluster, "enable out"=w245:bool, "axis"=w262:u8, "deviceHandle"=w284:i32)  [unwired: 4 in]
              n140 = local write "RT in move Signal 3"(w245) -> ()
              n141 = local write "RT in move 3"(w245) -> ()
              n142 = call "AMC_controlAQuadBInResolution.vi"("set"=FALSE, "error in"=w312, "axis"=w272, "deviceHandle"=w317) -> ("error out"=w241:errorcluster, "resolution out"=w256:i32, "axis"=w242:u8, "deviceHandle"=w243:i32)  [unwired: 4 in]
              n143 = local write "AquadB in res 1"(w256) -> ()
              n144 = call "AMC_controlAQuadBInResolution.vi"("set"=FALSE, "error in"=w279, "axis"=w262, "deviceHandle"=w284) -> ("error out"=w208:errorcluster, "resolution out"=w244:i32, "axis"=w209:u8, "deviceHandle"=w210:i32)  [unwired: 4 in]
              n145 = local write "AquadB in res 3"(w244) -> ()
              n146 = call "AMC_controlAQuadBInResolution.vi"("set"=FALSE, "error in"=w310, "axis"=w267, "deviceHandle"=w305) -> ("error out"=w211:errorcluster, "resolution out"=w250:i32, "axis"=w212:u8, "deviceHandle"=w213:i32)  [unwired: 4 in]
              n147 = local write "AquadB in res 2"(w250) -> ()
              n148 = call "AMC_controlAQuadBOut.vi"("set"=FALSE, "error in"=w211, "axis"=w212, "deviceHandle"=w213) -> ("error out"=w227:errorcluster, "enable out"=w200:bool, "axis"=w225:u8, "deviceHandle"=w223:i32)  [unwired: 4 in]
              n149 = local write "AquadB out 2"(w200) -> ()
              n150 = call "AMC_controlAQuadBOut.vi"("set"=FALSE, "error in"=w208, "axis"=w209, "deviceHandle"=w210) -> ("error out"=w218:errorcluster, "enable out"=w199:bool, "axis"=w220:u8, "deviceHandle"=w222:i32)  [unwired: 4 in]
              n151 = local write "AquadB out 3"(w199) -> ()
              n152 = call "AMC_controlAQuadBOut.vi"("set"=FALSE, "error in"=w241, "axis"=w242, "deviceHandle"=w243) -> ("error out"=w236:errorcluster, "enable out"=w201:bool, "axis"=w238:u8, "deviceHandle"=w240:i32)  [unwired: 4 in]
              n153 = local write "AquadB out 1"(w201) -> ()
              n154 = call "AMC_controlAQuadBOutClock.vi"("set"=FALSE, "error in"=w227, "axis"=w225, "deviceHandle"=w223) -> ("error out"=w228:errorcluster, "clock out"=w206:i32, "axis"=w226:u8, "deviceHandle"=w224:i32)  [unwired: 4 in]
              n155 = local write "AqaudB clock 2"(w206) -> ()
              n156 = call "AMC_controlAQuadBOutClock.vi"("set"=FALSE, "error in"=w218, "axis"=w220, "deviceHandle"=w222) -> ("error out"=w217:errorcluster, "clock out"=w205:i32, "axis"=w219:u8, "deviceHandle"=w221:i32)  [unwired: 4 in]
              n157 = local write "AqaudB clock 3"(w205) -> ()
              n158 = call "AMC_controlAQuadBOutClock.vi"("set"=FALSE, "error in"=w236, "axis"=w238, "deviceHandle"=w240) -> ("error out"=w235:errorcluster, "clock out"=w207:i32, "axis"=w237:u8, "deviceHandle"=w239:i32)  [unwired: 4 in]
              n159 = local write "AqaudB clock 1"(w207) -> ()
              n160 = call "AMC_controlAQuadBOutResolution.vi"("set"=FALSE, "error in"=w228, "axis"=w226, "deviceHandle"=w224) -> ("resolution out"=w203:i32)  [unwired: 4 in, 3 out]
              n161 = local write "AquadB Resolution 2"(w203) -> ()
              n162 = call "AMC_controlAQuadBOutResolution.vi"("set"=FALSE, "error in"=w217, "axis"=w219, "deviceHandle"=w221) -> ("resolution out"=w202:i32)  [unwired: 4 in, 3 out]
              n163 = local write "AquadB Resolution 3"(w202) -> ()
              n164 = call "AMC_controlAQuadBOutResolution.vi"("set"=FALSE, "error in"=w235, "axis"=w237, "deviceHandle"=w239) -> ("resolution out"=w204:i32)  [unwired: 4 in, 3 out]
              n165 = local write "AquadB Resolution 1"(w204) -> ()
            }
            frame #4 {
              n166 = disable-structure shown="Disabled" {
                disable-tunnel: w328 -> [w331 _]
                frame Disabled {
                  n167 = call "AMC_controlRtOutSignalMode.vi"("deviceHandle"=w331, "set"=FALSE) -> ("mode out"=w329:i32)  [unwired: 6 in, 2 out]
                  n168 = local write "Output Mode"(w329) -> ()
                }
                frame Enabled {
                }
              }
            }
          }
        }
        frame #1 {
          # "Main Loop"
          n169 = while {
            tunnel: w332 -> [w335]
            stop <- "stop" stop-if-true
            n170 = case shown="\"About\"" "Tab Control" {
              tunnel: w335 -> [w336 w919 w1305]
              frame "Navigation", Default {
                n171 = stacked-sequence {
                  tunnel: w336 -> [w343 w536 w730]
                  frame #0 {
                    w342 = u8 0 items=["1", "2", "3"] ("axis in")
                    n172 = event shown="[14] \"Target Range 1\": Value Change" {
                      selector: _ -> [_ _ _ _ _ _ _ _ _ _ _ _ _ _ _ _ _ _]
                      dyn-events: _ -> [_ _ _ _ _ _ _ _ _ _ _ _ _ _ _ _ _ _]
                      timeout: 1 -> [_ _ _ _ _ _ _ _ _ _ _ _ _ _ _ _ _ _]
                      tunnel: w343 -> [w348 w363 w375 w385 w394 w407 w410 w423 w428 w436 w446 w456 _ w469 w480 w484 w494 w526]
                      tunnel: w342 -> [w347 w364 w373 w384 w393 w406 w409 w421 w427 w434 w444 w457 _ w468 w479 w483 w493 w504]
                      tunnel: [w346 w359 w367 w379 w388 w396 w408 w416 w426 w431 w447 w451 _ w463 w473 _ w492 w503] -> w340
                      event "Amplitude [V]": Value Change {
                        n173 = event-data() -> ()  [unwired: 1 in, 1 out]
                        n174 = call "AMC_controlAmplitude.vi"("set"=TRUE, "amplitude [V] in"="Amplitude [V]", "axis"=w347, "deviceHandle"=w348) -> ("error out"=w352:errorcluster, "axis"=w349:u8, "deviceHandle"=w353:i32)  [unwired: 2 in, 1 out]
                        n175 = call "AMC_controlAmplitude.vi"("set"=FALSE, "error in"=w352, "axis"=w349, "deviceHandle"=w353) -> ("error out"=w346:errorcluster, "amplitude [V] out"=w350:dbl)  [unwired: 2 in, 2 out]
                        n176 = local write "Amplitude [V]"(w350) -> ()
                      }
                      event "Output": Value Change {
                        n177 = event-data() -> ()  [unwired: 1 in, 1 out]
                        n178 = call "AMC_controlOutput.vi"("set"=TRUE, "enable in"="Output", "axis"=w364, "deviceHandle"=w363) -> ("error out"=w360:errorcluster, "axis"=w361:u8, "deviceHandle"=w362:i32)  [unwired: 4 in, 1 out]
                        n179 = call "AMC_controlOutput.vi"("set"=FALSE, "error in"=w360, "axis"=w361, "deviceHandle"=w362) -> ("error out"=w359:errorcluster, "enable out"=→"Output Status 1":bool)  [unwired: 4 in, 2 out]
                      }
                      event "Frequency [Hz]": Value Change {
                        n180 = event-data() -> ()  [unwired: 1 in, 1 out]
                        n181 = call "AMC_controlFrequency.vi"("set"=TRUE, "frequency [Hz] in"="Frequency [Hz]", "axis"=w373, "deviceHandle"=w375) -> ("error out"=w370:errorcluster, "axis"=w366:u8, "deviceHandle"=w371:i32)  [unwired: 4 in, 1 out]
                        n182 = call "AMC_controlFrequency.vi"("set"=FALSE, "error in"=w370, "axis"=w366, "deviceHandle"=w371) -> ("error out"=w367:errorcluster, "frequency [Hz] out"=w368:dbl)  [unwired: 4 in, 2 out]
                        n183 = local write "Frequency [Hz]"(w368) -> ()
                      }
                      event "Move": Value Change {
                        n184 = event-data() -> ()  [unwired: 1 in, 1 out]
                        n185 = call "AMC_controlMove.vi"("set"=TRUE, "enable in"="Move", "axis"=w384, "deviceHandle"=w385) -> ("error out"=w380:errorcluster, "axis"=w381:u8, "deviceHandle"=w382:i32)  [unwired: 4 in, 1 out]
                        n186 = call "AMC_controlMove.vi"("set"=FALSE, "error in"=w380, "axis"=w381, "deviceHandle"=w382) -> ("error out"=w379:errorcluster, "enable out"=→"move out":bool)  [unwired: 4 in, 2 out]
                      }
                      event "EoT 1": Value Change {
                        n187 = event-data() -> ()  [unwired: 1 in, 1 out]
                        n188 = call "AMC_controlEotOutputDeactive.vi"("set"=TRUE, "enable in"="EoT 1", "axis"=w393, "deviceHandle"=w394) -> ("error out"=w390:errorcluster, "axis"=w391:u8, "deviceHandle"=w392:i32)  [unwired: 4 in, 1 out]
                        n189 = call "AMC_controlEotOutputDeactive.vi"("set"=FALSE, "error in"=w390, "axis"=w391, "deviceHandle"=w392) -> ("error out"=w388:errorcluster, "enable out"=w386:bool)  [unwired: 4 in, 2 out]
                        n190 = local write "EoT 1"(w386) -> ()
                      }
                      event "Target Position 1": Value Change {
                        n191 = event-data() -> ()  [unwired: 1 in, 1 out]
                        n192 = Multiply(x="Target Position 1", y=1000) -> (x*y=w402:i32)
                        n193 = call "AMC_controlTargetPosition.vi"("set"=TRUE, "target in"=w402, "axis"=w406, "deviceHandle"=w407) -> ("error out"=w399:errorcluster, "axis"=w400:u8, "deviceHandle"=w401:i32)  [unwired: 4 in, 1 out]
                        n194 = call "AMC_controlTargetPosition.vi"("set"=FALSE, "error in"=w399, "axis"=w400, "deviceHandle"=w401) -> ("error out"=w396:errorcluster, "target out"=w397:i32)  [unwired: 4 in, 2 out]
                        n195 = local write "Target Position 1"(w397) -> ()
                      }
                      event "Axis 1": Value Change {
                        n196 = event-data() -> ()  [unwired: 1 in, 1 out]
                        n197 = case shown="True" "Axis 1" {
                          tunnel: w410 -> [_ w413]
                          tunnel: w409 -> [_ w414]
                          tunnel: [_ w412] -> w408
                          frame False {
                          }
                          frame True {
                            n198 = call "AMC_setReset.vi"("axis"=w414, "deviceHandle"=w413) -> ("error out"=w412:errorcluster)  [unwired: 7 in, 2 out]
                          }
                        }
                      }
                      event "Single Step Left": Value Change {
                        n199 = event-data() -> ()  [unwired: 1 in, 1 out]
                        n200 = call "AMC_setNSteps.vi"("deviceHandle"=w423, "axis"=w421, "n in"="Number of steps 1", "backwards"=FALSE) -> ("deviceHandle"=w418:i32, "axis"=w417:i32, "error out"=w419:errorcluster)  [unwired: 8 in, 1 out]
                        n201 = call "AMC_getNSteps.vi"("error in"=w419, "axis"=w417, "deviceHandle"=w418) -> ("error out"=w416:errorcluster, "n out"=w415:i32)  [unwired: 5 in, 2 out]
                        n202 = local write "Number of steps 1"(w415) -> ()
                      }
                      event "Single Step Right": Value Change {
                        n203 = event-data() -> ()  [unwired: 1 in, 1 out]
                        n204 = local read "Number of steps 1"() -> (w424:i32)
                        n205 = call "AMC_setNSteps.vi"("deviceHandle"=w428, "axis"=w427, "n in"=w424, "backwards"=TRUE) -> ("error out"=w426:errorcluster)  [unwired: 8 in, 3 out]
                      }
                      event "Endless Left": Value Change {
                        n206 = event-data() -> ()  [unwired: 1 in, 1 out]
                        n207 = call "AMC_controlContinousFwd.vi"("set"=TRUE, "enable in"=FALSE, "axis"=w434, "deviceHandle"=w436) -> ("axis"=w433:u8, "deviceHandle"=w435:i32)  [unwired: 4 in, 2 out]
                        n208 = local write "Continuous Forward"(FALSE) -> ()
                        n209 = call "AMC_controlContinousBkwd.vi"("set"=TRUE, "enable in"="Endless Left", "axis"=w433, "deviceHandle"=w435) -> ("error out"=w431:errorcluster)  [unwired: 4 in, 3 out]
                      }
                      event "Continuous Forward": Value Change {
                        n210 = event-data() -> ()  [unwired: 1 in, 1 out]
                        n211 = call "AMC_controlContinousBkwd.vi"("set"=TRUE, "enable in"=FALSE, "axis"=w444, "deviceHandle"=w446) -> ("error out"=w442:errorcluster, "axis"=w443:u8, "deviceHandle"=w445:i32)  [unwired: 4 in, 1 out]
                        n212 = call "AMC_controlContinousFwd.vi"("set"=TRUE, "error in"=w442, "enable in"="Continuous Forward", "axis"=w443, "deviceHandle"=w445) -> ("error out"=w447:errorcluster)  [unwired: 3 in, 3 out]
                        n213 = local write "Endless Left"(FALSE) -> ()
                      }
                      event "Fixed DC 1": Value Change {
                        n214 = event-data() -> ()  [unwired: 1 in, 1 out]
                        n215 = call "AMC_controlFixOutputVoltage.vi"("set"=TRUE, "voltage"="Fixed DC 1", "axis"=w457, "deviceHandle"=w456) -> ("error out"=w452:errorcluster, "axis"=w454:u8, "deviceHandle"=w455:i32)  [unwired: 4 in, 1 out]
                        n216 = call "AMC_controlFixOutputVoltage.vi"("set"=FALSE, "error in"=w452, "axis"=w454, "deviceHandle"=w455) -> ("error out"=w451:errorcluster, "voltage"=w450:i32)  [unwired: 4 in, 2 out]
                        n217 = local write "Fixed DC 1"(w450) -> ()
                      }
                      event "Reset Error": Value Change {
                        n218 = event-data() -> ()  [unwired: 1 in, 1 out]
                        n219 = local write "Error Message"("" ("Error Message")) -> ()
                        n220 = local write "Error"(FALSE ("Error")) -> ()
                      }
                      event "Positioner": Value Change {
                        n221 = event-data() -> ()  [unwired: 1 in, 1 out]
                        n222 = property on="Positioner" class="Ring (strict)"() -> ("RingText.Text"=w467:string)  [unwired: 2 in, 2 out]
                        n223 = call "AMC_controlActorSelection.vi"("set"=TRUE, "actor in"=w467, "axis"=w468, "deviceHandle"=w469) -> ("error out"=w465:errorcluster, "axis"=w464:u8, "deviceHandle"=w466:i32)  [unwired: 4 in, 1 out]
                        n224 = call "AMC_getActorType.vi"("error in"=w465, "axis"=w464, "deviceHandle"=w466) -> ("error out"=w463:errorcluster, "positioner type"=→"actor type":u16)  [unwired: 5 in, 2 out]
                      }
                      event "Target Range 1": Value Change {
                        n225 = event-data() -> ()  [unwired: 1 in, 1 out]
                        n226 = call "AMC_controlTargetRange.vi"("set"=TRUE, "range in"="Target Range 1", "axis"=w479, "deviceHandle"=w480) -> ("error out"=w474:errorcluster, "axis"=w475:u8, "deviceHandle"=w476:i32)  [unwired: 4 in, 1 out]
                        n227 = call "AMC_controlTargetRange.vi"("set"=FALSE, "error in"=w474, "axis"=w475, "deviceHandle"=w476) -> ("error out"=w473:errorcluster, "range out"=w471:u32)  [unwired: 4 in, 2 out]
                        n228 = local write "Target Range 1"(w471) -> ()
                      }
                      event "auto Reset 1": Value Change {
                        n229 = event-data() -> ()  [unwired: 1 in, 1 out]
                        n230 = call "AMC_controlAutoReset.vi"("set"=TRUE, "enable in"="auto Reset 1", "axis"=w483, "deviceHandle in"=w484) -> ("error out"=w488:errorcluster, "axis"=w487:u8, "deviceHandle out"=w486:i32)  [unwired: 4 in, 1 out]
                        n231 = call "AMC_controlAutoReset.vi"("set"=FALSE, "error in"=w488, "axis"=w487, "deviceHandle in"=w486) -> ("enable out"=w481:bool)  [unwired: 4 in, 3 out]
                        n232 = local write "auto Reset 1"(w481) -> ()
                      }
                      event "Reference Auto Update 3": Value Change {
                        n233 = event-data() -> ()  [unwired: 1 in, 1 out]
                        n234 = call "AMC_controlReferenceAutoUpdate.vi"("set"=TRUE, "enable in"="Reference Auto Update 1", "axis"=w493, "deviceHandle"=w494) -> ("error out"=w496:errorcluster, "axis"=w498:u8, "deviceHandle"=w497:i32)  [unwired: 4 in, 1 out]
                        n235 = call "AMC_controlReferenceAutoUpdate.vi"("set"=FALSE, "error in"=w496, "axis"=w498, "deviceHandle"=w497) -> ("error out"=w492:errorcluster, "enable out"=w490:bool)  [unwired: 4 in, 2 out]
                        n236 = local write "Reference Auto Update 1"(w490) -> ()
                      }
                      event Timeout {
                        n237 = event-data() -> ()  [unwired: 1 in, 1 out]
                        n238 = call "AMC_getPosition.vi"("axis"=w504, "deviceHandle"=w526) -> ("error out"=w525:errorcluster, "position"=→"Position":i32, "axis"=w518:u8, "deviceHandle"=w519:i32)  [unwired: 6 in]
                        n239 = call "AMC_getReferencePosition.vi"("error in"=w525, "axis"=w518, "deviceHandle"=w519) -> ("error out"=w513:errorcluster, "reference"=→"Reference":i32, "axis"=w515:i32, "deviceHandle"=w517:i32)  [unwired: 5 in]
                        n240 = call "AMC_getStatusConnected.vi"("error in"=w513, "axis"=w515, "deviceHandle"=w517) -> ("error out"=w512:errorcluster, "connected"=→"Connected":bool, "axis"=w514:i32, "deviceHandle"=w516:i32)  [unwired: 5 in]
                        n241 = call "AMC_getStatusMoving.vi"("error in"=w512, "axis"=w514, "deviceHandle"=w516) -> ("error out"=w530:errorcluster, "moving"=→"MoveSignal":bool, "axis"=w527:i32, "deviceHandle"=w531:i32)  [unwired: 5 in]
                        n242 = call "AMC_getStatusReference.vi"("error in"=w530, "axis"=w527, "deviceHandle"=w531) -> ("error out"=w505:errorcluster, "reference valid"=→"ReferenceSignal":bool, "axis"=w506:i32, "deviceHandle"=w507:i32)  [unwired: 5 in]
                        n243 = call "AMC_getStatusEotBkwd.vi"("error in"=w505, "axis"=w506, "deviceHandle"=w507) -> ("error out"=w523:errorcluster, "EotDetected"=→"EotLeftDetected1":bool, "axis"=w521:u8, "deviceHandle"=w522:i32)  [unwired: 5 in]
                        n244 = call "AMC_getStatusEotFwd.vi"("error in"=w523, "axis"=w521, "deviceHandle"=w522) -> ("error out"=w508:errorcluster, "EotDetected"=→"EotrightDetected1":bool, "axis"=w509:u8, "deviceHandle"=w510:i32)  [unwired: 5 in]
                        n245 = call "AMC_getStatusTargetRange.vi"("error in"=w508, "axis"=w509, "deviceHandle"=w510) -> ("error out"=w503:errorcluster, "in target range"=→"in target range1":bool)  [unwired: 5 in, 2 out]
                      }
                    }
                    n246 = Unbundle(w340) -> ("code"=w338:i32, "source"=w339:string)  [unwired: 1 out]
                    n247 = Not Equal To 0?(x=w338) -> (x != 0?=w337:bool)
                    n248 = case shown="True" w337 {
                      selector: w337 -> [_ w344]
                      tunnel: w339 -> [_ w345]
                      frame False {
                      }
                      frame True {
                        "Error Message" <- w345
                        "Error" <- w344
                      }
                    }
                  }
                  frame #1 {
                    w538 = u8 1 items=["1", "2", "3"] ("axis in")
                    n249 = event shown="[3] \"Move 2\": Value Change" {
                      selector: _ -> [_ _ _ _ _ _ _ _ _ _ _ _ _ _ _ _ _ _]
                      dyn-events: _ -> [_ _ _ _ _ _ _ _ _ _ _ _ _ _ _ _ _ _]
                      timeout: 1 -> [_ _ _ _ _ _ _ _ _ _ _ _ _ _ _ _ _ _]
                      tunnel: w536 -> [w550 w560 w570 w580 w589 w602 w606 w618 w623 w630 w642 w652 _ w665 w675 w679 w688 w718]
                      tunnel: w538 -> [w549 w559 w569 w579 w588 w600 w605 w617 w622 w629 w640 w653 _ w664 w674 w678 w687 w717]
                      tunnel: [w544 w553 w564 w574 w583 w593 w603 w610 w621 w632 w643 w648 _ w659 _ _ _ w700] -> w534
                      event "amplitude [V] 2": Value Change {
                        n250 = event-data() -> ()  [unwired: 1 in, 1 out]
                        n251 = call "AMC_controlAmplitude.vi"("set"=TRUE, "amplitude [V] in"="amplitude [V] 2", "axis"=w549, "deviceHandle"=w550) -> ("error out"=w545:errorcluster, "axis"=w541:u8, "deviceHandle"=w546:i32)  [unwired: 2 in, 1 out]
                        n252 = call "AMC_controlAmplitude.vi"("set"=FALSE, "error in"=w545, "axis"=w541, "deviceHandle"=w546) -> ("error out"=w544:errorcluster, "amplitude [V] out"=w542:dbl)  [unwired: 2 in, 2 out]
                        n253 = local write "amplitude [V] 2"(w542) -> ()
                      }
                      event "Output 2": Value Change {
                        n254 = event-data() -> ()  [unwired: 1 in, 1 out]
                        n255 = call "AMC_controlOutput.vi"("set"=TRUE, "enable in"="Output 2", "axis"=w559, "deviceHandle"=w560) -> ("error out"=w555:errorcluster, "axis"=w556:u8, "deviceHandle"=w557:i32)  [unwired: 4 in, 1 out]
                        n256 = call "AMC_controlOutput.vi"("set"=FALSE, "error in"=w555, "axis"=w556, "deviceHandle"=w557) -> ("error out"=w553:errorcluster, "enable out"=→"Output Status 2":bool)  [unwired: 4 in, 2 out]
                      }
                      event "frequency [Hz] 2": Value Change {
                        n257 = event-data() -> ()  [unwired: 1 in, 1 out]
                        n258 = call "AMC_controlFrequency.vi"("set"=TRUE, "frequency [Hz] in"="frequency [Hz] 2", "axis"=w569, "deviceHandle"=w570) -> ("error out"=w565:errorcluster, "axis"=w561:u8, "deviceHandle"=w566:i32)  [unwired: 4 in, 1 out]
                        n259 = call "AMC_controlFrequency.vi"("set"=FALSE, "error in"=w565, "axis"=w561, "deviceHandle"=w566) -> ("error out"=w564:errorcluster, "frequency [Hz] out"=w562:dbl)  [unwired: 4 in, 2 out]
                        n260 = local write "frequency [Hz] 2"(w562) -> ()
                      }
                      event "Move 2": Value Change {
                        n261 = event-data() -> ()  [unwired: 1 in, 1 out]
                        n262 = call "AMC_controlMove.vi"("set"=TRUE, "enable in"="Move 2", "axis"=w579, "deviceHandle"=w580) -> ("error out"=w575:errorcluster, "axis"=w576:u8, "deviceHandle"=w577:i32)  [unwired: 4 in, 1 out]
                        n263 = call "AMC_controlMove.vi"("set"=FALSE, "error in"=w575, "axis"=w576, "deviceHandle"=w577) -> ("error out"=w574:errorcluster, "enable out"=→"move out 2":bool)  [unwired: 4 in, 2 out]
                      }
                      event "EoT 2": Value Change {
                        n264 = event-data() -> ()  [unwired: 1 in, 1 out]
                        n265 = call "AMC_controlEotOutputDeactive.vi"("set"=TRUE, "enable in"="EoT 2", "axis"=w588, "deviceHandle"=w589) -> ("error out"=w585:errorcluster, "axis"=w586:u8, "deviceHandle"=w587:i32)  [unwired: 4 in, 1 out]
                        n266 = call "AMC_controlEotOutputDeactive.vi"("set"=FALSE, "error in"=w585, "axis"=w586, "deviceHandle"=w587) -> ("error out"=w583:errorcluster, "enable out"=w581:bool)  [unwired: 4 in, 2 out]
                        n267 = local write "EoT 2"(w581) -> ()
                      }
                      event "Target position 2": Value Change {
                        n268 = event-data() -> ()  [unwired: 1 in, 1 out]
                        n269 = Multiply(x="Target position 2", y=1000) -> (x*y=w598:i32)
                        n270 = call "AMC_controlTargetPosition.vi"("set"=TRUE, "target in"=w598, "axis"=w600, "deviceHandle"=w602) -> ("error out"=w595:errorcluster, "axis"=w594:u8, "deviceHandle"=w596:i32)  [unwired: 4 in, 1 out]
                        n271 = call "AMC_controlTargetPosition.vi"("set"=FALSE, "error in"=w595, "axis"=w594, "deviceHandle"=w596) -> ("error out"=w593:errorcluster, "target out"=w592:i32)  [unwired: 4 in, 2 out]
                        n272 = local write "Target position 2"(w592) -> ()
                      }
                      event "Axis 2": Value Change {
                        n273 = event-data() -> ()  [unwired: 1 in, 1 out]
                        n274 = case shown="True" "Axis 2" {
                          tunnel: w606 -> [_ w608]
                          tunnel: w605 -> [_ w609]
                          tunnel: [_ w607] -> w603
                          frame False {
                          }
                          frame True {
                            n275 = call "AMC_setReset.vi"("axis"=w609, "deviceHandle"=w608) -> ("error out"=w607:errorcluster)  [unwired: 7 in, 2 out]
                          }
                        }
                      }
                      event "Single Step Left 2": Value Change {
                        n276 = event-data() -> ()  [unwired: 1 in, 1 out]
                        n277 = call "AMC_setNSteps.vi"("deviceHandle"=w618, "axis"=w617, "n in"="Number of steps 2", "backwards"=FALSE) -> ("deviceHandle"=w613:i32, "axis"=w612:i32, "error out"=w614:errorcluster)  [unwired: 8 in, 1 out]
                        n278 = call "AMC_getNSteps.vi"("error in"=w614, "axis"=w612, "deviceHandle"=w613) -> ("error out"=w610:errorcluster, "n out"=w611:i32)  [unwired: 5 in, 2 out]
                        n279 = local write "Number of steps 2"(w611) -> ()
                      }
                      event "Single Step Right 2": Value Change {
                        n280 = event-data() -> ()  [unwired: 1 in, 1 out]
                        n281 = local read "Number of steps 2"() -> (w619:i32)
                        n282 = call "AMC_setNSteps.vi"("deviceHandle"=w623, "axis"=w622, "n in"=w619, "backwards"=TRUE) -> ("error out"=w621:errorcluster)  [unwired: 8 in, 3 out]
                      }
                      event "Endless Left 2": Value Change {
                        n283 = event-data() -> ()  [unwired: 1 in, 1 out]
                        n284 = call "AMC_controlContinousFwd.vi"("set"=TRUE, "enable in"=FALSE, "axis"=w629, "deviceHandle"=w630) -> ("error out"=w627:errorcluster, "axis"=w628:u8, "deviceHandle"=w631:i32)  [unwired: 4 in, 1 out]
                        n285 = call "AMC_controlContinousBkwd.vi"("set"=TRUE, "error in"=w627, "enable in"="Endless Left 2", "axis"=w628, "deviceHandle"=w631) -> ("error out"=w632:errorcluster)  [unwired: 3 in, 3 out]
                        n286 = local write "Continuous Forward"(FALSE) -> ()
                      }
                      event "Continuous Forward": Value Change {
                        n287 = event-data() -> ()  [unwired: 1 in, 1 out]
                        n288 = call "AMC_controlContinousBkwd.vi"("set"=TRUE, "enable in"=FALSE, "axis"=w640, "deviceHandle"=w642) -> ("error out"=w638:errorcluster, "axis"=w639:u8, "deviceHandle"=w641:i32)  [unwired: 4 in, 1 out]
                        n289 = call "AMC_controlContinousFwd.vi"("set"=TRUE, "error in"=w638, "enable in"="Continuous Forward", "axis"=w639, "deviceHandle"=w641) -> ("error out"=w643:errorcluster)  [unwired: 3 in, 3 out]
                        n290 = local write "Endless Left 2"(FALSE ("Endless Left 2")) -> ()
                      }
                      event "Fixed DC 2": Value Change {
                        n291 = event-data() -> ()  [unwired: 1 in, 1 out]
                        n292 = call "AMC_controlFixOutputVoltage.vi"("set"=TRUE, "voltage"="Fixed DC 2", "axis"=w653, "deviceHandle"=w652) -> ("error out"=w649:errorcluster, "axis"=w650:u8, "deviceHandle"=w651:i32)  [unwired: 4 in, 1 out]
                        n293 = call "AMC_controlFixOutputVoltage.vi"("set"=FALSE, "error in"=w649, "axis"=w650, "deviceHandle"=w651) -> ("error out"=w648:errorcluster, "voltage"=w646:i32)  [unwired: 4 in, 2 out]
                        n294 = local write "Fixed DC 2"(w646) -> ()
                      }
                      event "Reset Error 2": Value Change {
                        n295 = event-data() -> ()  [unwired: 1 in, 1 out]
                        n296 = local write "Error Message 2"("" ("Error Message 2")) -> ()
                        n297 = local write "Error 2"(FALSE ("Error 2")) -> ()
                      }
                      event "Positioner 2": Value Change {
                        n298 = event-data() -> ()  [unwired: 1 in, 1 out]
                        n299 = property on="Positioner 2" class="Ring (strict)"() -> ("RingText.Text"=w663:string)  [unwired: 2 in, 2 out]
                        n300 = call "AMC_controlActorSelection.vi"("set"=TRUE, "actor in"=w663, "axis"=w664, "deviceHandle"=w665) -> ("error out"=w660:errorcluster, "axis"=w661:u8, "deviceHandle"=w662:i32)  [unwired: 4 in, 1 out]
                        n301 = call "AMC_getActorType.vi"("error in"=w660, "axis"=w661, "deviceHandle"=w662) -> ("error out"=w659:errorcluster, "positioner type"=→"actor type 2":u16)  [unwired: 5 in, 2 out]
                      }
                      event "Target Range 2": Value Change {
                        n302 = event-data() -> ()  [unwired: 1 in, 1 out]
                        n303 = call "AMC_controlTargetRange.vi"("set"=TRUE, "range in"="Target Range 2", "axis"=w674, "deviceHandle"=w675) -> ("error out"=w669:errorcluster, "axis"=w670:u8, "deviceHandle"=w671:i32)  [unwired: 4 in, 1 out]
                        n304 = call "AMC_controlTargetRange.vi"("set"=FALSE, "error in"=w669, "axis"=w670, "deviceHandle"=w671) -> ("range out"=w667:u32)  [unwired: 4 in, 3 out]
                        n305 = local write "Target Range 2"(w667) -> ()
                      }
                      event "auto Reset 2": Value Change {
                        n306 = event-data() -> ()  [unwired: 1 in, 1 out]
                        n307 = call "AMC_controlAutoReset.vi"("set"=TRUE, "enable in"="auto Reset 2", "axis"=w678, "deviceHandle in"=w679) -> ("error out"=w683:errorcluster, "axis"=w682:u8, "deviceHandle out"=w681:i32)  [unwired: 4 in, 1 out]
                        n308 = call "AMC_controlAutoReset.vi"("set"=FALSE, "error in"=w683, "axis"=w682, "deviceHandle in"=w681) -> ("enable out"=w676:bool)  [unwired: 4 in, 3 out]
                        n309 = local write "auto Reset 2"(w676) -> ()
                      }
                      event "Reference Auto Update 2": Value Change {
                        n310 = event-data() -> ()  [unwired: 1 in, 1 out]
                        n311 = call "AMC_controlReferenceAutoUpdate.vi"("set"=TRUE, "enable in"="Reference Auto Update 2", "axis"=w687, "deviceHandle"=w688) -> ("error out"=w690:errorcluster, "axis"=w692:u8, "deviceHandle"=w691:i32)  [unwired: 4 in, 1 out]
                        n312 = call "AMC_controlReferenceAutoUpdate.vi"("set"=FALSE, "error in"=w690, "axis"=w692, "deviceHandle"=w691) -> ("enable out"=w685:bool)  [unwired: 4 in, 3 out]
                        n313 = local write "Reference Auto Update 2"(w685) -> ()
                      }
                      event Timeout {
                        n314 = event-data() -> ()  [unwired: 1 in, 1 out]
                        n315 = call "AMC_getPosition.vi"("axis"=w717, "deviceHandle"=w718) -> ("error out"=w716:errorcluster, "position"=→"Position 2":i32, "axis"=w722:u8, "deviceHandle"=w723:i32)  [unwired: 6 in]
                        n316 = call "AMC_getReferencePosition.vi"("error in"=w716, "axis"=w722, "deviceHandle"=w723) -> ("error out"=w706:errorcluster, "reference"=→"Reference 2":i32, "axis"=w708:i32, "deviceHandle"=w710:i32)  [unwired: 5 in]
                        n317 = call "AMC_getStatusConnected.vi"("error in"=w706, "axis"=w708, "deviceHandle"=w710) -> ("error out"=w705:errorcluster, "connected"=→"Connected 2":bool, "axis"=w707:i32, "deviceHandle"=w709:i32)  [unwired: 5 in]
                        n318 = call "AMC_getStatusMoving.vi"("error in"=w705, "axis"=w707, "deviceHandle"=w709) -> ("error out"=w724:errorcluster, "moving"=→"MoveSignal 2":bool, "axis"=w719:i32, "deviceHandle"=w725:i32)  [unwired: 5 in]
                        n319 = call "AMC_getStatusReference.vi"("error in"=w724, "axis"=w719, "deviceHandle"=w725) -> ("error out"=w697:errorcluster, "reference valid"=→"ReferenceSignal 2":bool, "axis"=w698:i32, "deviceHandle"=w699:i32)  [unwired: 5 in]
                        n320 = call "AMC_getStatusEotBkwd.vi"("error in"=w697, "axis"=w698, "deviceHandle"=w699) -> ("error out"=w712:errorcluster, "EotDetected"=→"EotLeftDetected2":bool, "axis"=w713:u8, "deviceHandle"=w714:i32)  [unwired: 5 in]
                        n321 = call "AMC_getStatusEotFwd.vi"("error in"=w712, "axis"=w713, "deviceHandle"=w714) -> ("error out"=w701:errorcluster, "EotDetected"=→"EotrightDetected2":bool, "axis"=w702:u8, "deviceHandle"=w703:i32)  [unwired: 5 in]
                        n322 = call "AMC_getStatusTargetRange.vi"("error in"=w701, "axis"=w702, "deviceHandle"=w703) -> ("error out"=w700:errorcluster, "in target range"=→"in target range2":bool)  [unwired: 5 in, 2 out]
                      }
                    }
                    n323 = Unbundle(w534) -> ("code"=w533:i32, "source"=w535:string)  [unwired: 1 out]
                    n324 = Not Equal To 0?(x=w533) -> (x != 0?=w532:bool)
                    n325 = case shown="True" w532 {
                      selector: w532 -> [_ w539]
                      tunnel: w535 -> [_ w540]
                      frame False {
                      }
                      frame True {
                        "Error Message 2" <- w540
                        "Error 2" <- w539
                      }
                    }
                  }
                  frame #2 {
                    w732 = u8 2 items=["1", "2", "3"] ("axis in")
                    n326 = event shown="[7] \"Single Step Left 3\": Value Change" {
                      selector: _ -> [_ _ _ _ _ _ _ _ _ _ _ _ _ _ _ _ _ _]
                      dyn-events: _ -> [_ _ _ _ _ _ _ _ _ _ _ _ _ _ _ _ _ _]
                      timeout: 1 -> [_ _ _ _ _ _ _ _ _ _ _ _ _ _ _ _ _ _]
                      tunnel: w730 -> [w744 w753 w764 w774 w783 w796 w800 w811 w816 w823 w834 w844 _ w857 w867 w872 w881 w911]
                      tunnel: w732 -> [w743 w752 w763 w773 w782 w795 w799 w810 w815 w821 w832 w845 _ w856 w866 w871 w880 w910]
                      tunnel: [w738 w747 w758 w770 w777 w787 w797 _ w814 w824 w835 w839 _ w851 w861 _ _ w893] -> w728
                      event "amplitude [V] 3": Value Change {
                        n327 = event-data() -> ()  [unwired: 1 in, 1 out]
                        n328 = call "AMC_controlAmplitude.vi"("set"=TRUE, "amplitude [V] in"="amplitude [V] 3", "axis"=w743, "deviceHandle"=w744) -> ("error out"=w739:errorcluster, "axis"=w735:u8, "deviceHandle"=w740:i32)  [unwired: 2 in, 1 out]
                        n329 = call "AMC_controlAmplitude.vi"("set"=FALSE, "error in"=w739, "axis"=w735, "deviceHandle"=w740) -> ("error out"=w738:errorcluster, "amplitude [V] out"=w736:dbl)  [unwired: 2 in, 2 out]
                        n330 = local write "amplitude [V] 3"(w736) -> ()
                      }
                      event "Output 3": Value Change {
                        n331 = event-data() -> ()  [unwired: 1 in, 1 out]
                        n332 = call "AMC_controlOutput.vi"("set"=TRUE, "enable in"="Output 3", "axis"=w752, "deviceHandle"=w753) -> ("error out"=w749:errorcluster, "axis"=w750:u8, "deviceHandle"=w751:i32)  [unwired: 4 in, 1 out]
                        n333 = call "AMC_controlOutput.vi"("set"=FALSE, "error in"=w749, "axis"=w750, "deviceHandle"=w751) -> ("error out"=w747:errorcluster, "enable out"=→"Output Status 3":bool)  [unwired: 4 in, 2 out]
                      }
                      event "frequency [Hz] 3": Value Change {
                        n334 = event-data() -> ()  [unwired: 1 in, 1 out]
                        n335 = call "AMC_controlFrequency.vi"("set"=TRUE, "frequency [Hz] in"="frequency [Hz] 3", "axis"=w763, "deviceHandle"=w764) -> ("error out"=w759:errorcluster, "axis"=w755:u8, "deviceHandle"=w760:i32)  [unwired: 4 in, 1 out]
                        n336 = call "AMC_controlFrequency.vi"("set"=FALSE, "error in"=w759, "axis"=w755, "deviceHandle"=w760) -> ("error out"=w758:errorcluster, "frequency [Hz] out"=w757:dbl)  [unwired: 4 in, 2 out]
                        n337 = local write "frequency [Hz] 3"(w757) -> ()
                      }
                      event "Move 3": Value Change {
                        n338 = event-data() -> ()  [unwired: 1 in, 1 out]
                        n339 = call "AMC_controlMove.vi"("set"=TRUE, "enable in"="Move 3", "axis"=w773, "deviceHandle"=w774) -> ("error out"=w771:errorcluster, "axis"=w768:u8, "deviceHandle"=w769:i32)  [unwired: 4 in, 1 out]
                        n340 = call "AMC_controlMove.vi"("set"=FALSE, "error in"=w771, "axis"=w768, "deviceHandle"=w769) -> ("error out"=w770:errorcluster, "enable out"=→"move out 3":bool)  [unwired: 4 in, 2 out]
                      }
                      event "EoT 3": Value Change {
                        n341 = event-data() -> ()  [unwired: 1 in, 1 out]
                        n342 = call "AMC_controlEotOutputDeactive.vi"("set"=TRUE, "enable in"="EoT 3", "axis"=w782, "deviceHandle"=w783) -> ("error out"=w779:errorcluster, "axis"=w780:u8, "deviceHandle"=w781:i32)  [unwired: 4 in, 1 out]
                        n343 = call "AMC_controlEotOutputDeactive.vi"("set"=FALSE, "error in"=w779, "axis"=w780, "deviceHandle"=w781) -> ("error out"=w777:errorcluster, "enable out"=w775:bool)  [unwired: 4 in, 2 out]
                        n344 = local write "EoT 3"(w775) -> ()
                      }
                      event "Target Position 3": Value Change {
                        n345 = event-data() -> ()  [unwired: 1 in, 1 out]
                        n346 = Multiply(x="Target Position 3", y=1000) -> (x*y=w791:i32)
                        n347 = call "AMC_controlTargetPosition.vi"("set"=TRUE, "target in"=w791, "axis"=w795, "deviceHandle"=w796) -> ("error out"=w788:errorcluster, "axis"=w789:u8, "deviceHandle"=w790:i32)  [unwired: 4 in, 1 out]
                        n348 = call "AMC_controlTargetPosition.vi"("set"=FALSE, "error in"=w788, "axis"=w789, "deviceHandle"=w790) -> ("error out"=w787:errorcluster, "target out"=w785:i32)  [unwired: 4 in, 2 out]
                        n349 = local write "Target Position 3"(w785) -> ()
                      }
                      event "Axis 3": Value Change {
                        n350 = event-data() -> ()  [unwired: 1 in, 1 out]
                        n351 = case shown="True" "Axis 3" {
                          tunnel: w800 -> [_ w802]
                          tunnel: w799 -> [_ w803]
                          tunnel: [_ w801] -> w797
                          frame False {
                          }
                          frame True {
                            n352 = call "AMC_setReset.vi"("axis"=w803, "deviceHandle"=w802) -> ("error out"=w801:errorcluster)  [unwired: 7 in, 2 out]
                          }
                        }
                      }
                      event "Single Step Left 3": Value Change {
                        n353 = event-data() -> ()  [unwired: 1 in, 1 out]
                        n354 = call "AMC_setNSteps.vi"("deviceHandle"=w811, "axis"=w810, "n in"="Number of steps 3", "backwards"=FALSE) -> ("deviceHandle"=w807:i32, "axis"=w806:i32, "error out"=w805:errorcluster)  [unwired: 8 in, 1 out]
                        n355 = call "AMC_getNSteps.vi"("error in"=w805, "axis"=w806, "deviceHandle"=w807) -> ("n out"=w804:i32)  [unwired: 5 in, 3 out]
                        n356 = local write "Number of steps 3"(w804) -> ()
                      }
                      event "Single Step Right 3": Value Change {
                        n357 = event-data() -> ()  [unwired: 1 in, 1 out]
                        n358 = local read "Number of steps 3"() -> (w812:i32)
                        n359 = call "AMC_setNSteps.vi"("deviceHandle"=w816, "axis"=w815, "n in"=w812, "backwards"=TRUE) -> ("error out"=w814:errorcluster)  [unwired: 8 in, 3 out]
                      }
                      event "Endless Left 3": Value Change {
                        n360 = event-data() -> ()  [unwired: 1 in, 1 out]
                        n361 = call "AMC_controlContinousFwd.vi"("set"=TRUE, "enable in"=FALSE, "axis"=w821, "deviceHandle"=w823) -> ("axis"=w820:u8, "deviceHandle"=w822:i32)  [unwired: 4 in, 2 out]
                        n362 = call "AMC_controlContinousBkwd.vi"("set"=TRUE, "enable in"="Endless Left 3", "axis"=w820, "deviceHandle"=w822) -> ("error out"=w824:errorcluster)  [unwired: 4 in, 3 out]
                        n363 = local write "Continuous Forward"(FALSE ("Endless Right 3")) -> ()
                      }
                      event "Continuous Forward": Value Change {
                        n364 = event-data() -> ()  [unwired: 1 in, 1 out]
                        n365 = call "AMC_controlContinousBkwd.vi"("set"=TRUE, "enable in"=FALSE, "axis"=w832, "deviceHandle"=w834) -> ("error out"=w830:errorcluster, "axis"=w831:u8, "deviceHandle"=w833:i32)  [unwired: 4 in, 1 out]
                        n366 = call "AMC_controlContinousFwd.vi"("set"=TRUE, "error in"=w830, "enable in"="Continuous Forward", "axis"=w831, "deviceHandle"=w833) -> ("error out"=w835:errorcluster)  [unwired: 3 in, 3 out]
                        n367 = local write "Endless Left 3"(FALSE ("Endless Left 3")) -> ()
                      }
                      event "Fixed DC 3": Value Change {
                        n368 = event-data() -> ()  [unwired: 1 in, 1 out]
                        n369 = call "AMC_controlFixOutputVoltage.vi"("set"=TRUE, "voltage"="Fixed DC 3", "axis"=w845, "deviceHandle"=w844) -> ("error out"=w841:errorcluster, "axis"=w842:u8, "deviceHandle"=w843:i32)  [unwired: 4 in, 1 out]
                        n370 = call "AMC_controlFixOutputVoltage.vi"("set"=FALSE, "error in"=w841, "axis"=w842, "deviceHandle"=w843) -> ("error out"=w839:errorcluster, "voltage"=w838:i32)  [unwired: 4 in, 2 out]
                        n371 = local write "Fixed DC 3"(w838) -> ()
                      }
                      event "Reset Error 3": Value Change {
                        n372 = event-data() -> ()  [unwired: 1 in, 1 out]
                        n373 = local write "Error Message 3"("" ("Error Message 3")) -> ()
                        n374 = local write "Error 3"(FALSE ("Error 3")) -> ()
                      }
                      event "Positioner 3": Value Change {
                        n375 = event-data() -> ()  [unwired: 1 in, 1 out]
                        n376 = property on="Positioner 3" class="Ring (strict)"() -> ("RingText.Text"=w855:string)  [unwired: 2 in, 2 out]
                        n377 = call "AMC_controlActorSelection.vi"("set"=TRUE, "actor in"=w855, "axis"=w856, "deviceHandle"=w857) -> ("error out"=w853:errorcluster, "axis"=w852:u8, "deviceHandle"=w854:i32)  [unwired: 4 in, 1 out]
                        n378 = call "AMC_getActorType.vi"("error in"=w853, "axis"=w852, "deviceHandle"=w854) -> ("error out"=w851:errorcluster, "positioner type"=→"actor type 3":u16)  [unwired: 5 in, 2 out]
                      }
                      event "Target Range 3": Value Change {
                        n379 = event-data() -> ()  [unwired: 1 in, 1 out]
                        n380 = call "AMC_controlTargetRange.vi"("set"=TRUE, "range in"="Target Range 3", "axis"=w866, "deviceHandle"=w867) -> ("error out"=w862:errorcluster, "axis"=w863:u8, "deviceHandle"=w864:i32)  [unwired: 4 in, 1 out]
                        n381 = call "AMC_controlTargetRange.vi"("set"=FALSE, "error in"=w862, "axis"=w863, "deviceHandle"=w864) -> ("error out"=w861:errorcluster, "range out"=w859:u32)  [unwired: 4 in, 2 out]
                        n382 = local write "Target Range 3"(w859) -> ()
                      }
                      event "auto Reset 3": Value Change {
                        n383 = event-data() -> ()  [unwired: 1 in, 1 out]
                        n384 = call "AMC_controlAutoReset.vi"("set"=TRUE, "enable in"="auto Reset 3", "axis"=w871, "deviceHandle in"=w872) -> ("error out"=w874:errorcluster, "axis"=w875:u8, "deviceHandle out"=w876:i32)  [unwired: 4 in, 1 out]
                        n385 = call "AMC_controlAutoReset.vi"("set"=FALSE, "error in"=w874, "axis"=w875, "deviceHandle in"=w876) -> ("enable out"=w869:bool)  [unwired: 4 in, 3 out]
                        n386 = local write "auto Reset 3"(w869) -> ()
                      }
                      event "Reference Auto Update 3": Value Change {
                        n387 = event-data() -> ()  [unwired: 1 in, 1 out]
                        n388 = call "AMC_controlReferenceAutoUpdate.vi"("set"=TRUE, "enable in"="Reference Auto Update 3", "axis"=w880, "deviceHandle"=w881) -> ("error out"=w885:errorcluster, "axis"=w883:u8, "deviceHandle"=w884:i32)  [unwired: 4 in, 1 out]
                        n389 = call "AMC_controlReferenceAutoUpdate.vi"("set"=FALSE, "error in"=w885, "axis"=w883, "deviceHandle"=w884) -> ("enable out"=w878:bool)  [unwired: 4 in, 3 out]
                        n390 = local write "Reference Auto Update 3"(w878) -> ()
                      }
                      event Timeout {
                        n391 = event-data() -> ()  [unwired: 1 in, 1 out]
                        n392 = call "AMC_getPosition.vi"("axis"=w910, "deviceHandle"=w911) -> ("error out"=w909:errorcluster, "position"=→"Position 3":i32, "axis"=w915:u8, "deviceHandle"=w916:i32)  [unwired: 6 in]
                        n393 = call "AMC_getReferencePosition.vi"("error in"=w909, "axis"=w915, "deviceHandle"=w916) -> ("error out"=w899:errorcluster, "reference"=→"Reference 3":i32, "axis"=w901:i32, "deviceHandle"=w903:i32)  [unwired: 5 in]
                        n394 = call "AMC_getStatusConnected.vi"("error in"=w899, "axis"=w901, "deviceHandle"=w903) -> ("error out"=w898:errorcluster, "connected"=→"Connected 3":bool, "axis"=w900:i32, "deviceHandle"=w902:i32)  [unwired: 5 in]
                        n395 = call "AMC_getStatusMoving.vi"("error in"=w898, "axis"=w900, "deviceHandle"=w902) -> ("error out"=w917:errorcluster, "moving"=→"MoveSignal 3":bool, "axis"=w912:i32, "deviceHandle"=w918:i32)  [unwired: 5 in]
                        n396 = call "AMC_getStatusReference.vi"("error in"=w917, "axis"=w912, "deviceHandle"=w918) -> ("error out"=w890:errorcluster, "reference valid"=→"ReferenceSignal 3":bool, "axis"=w891:i32, "deviceHandle"=w892:i32)  [unwired: 5 in]
                        n397 = call "AMC_getStatusEotBkwd.vi"("error in"=w890, "axis"=w891, "deviceHandle"=w892) -> ("error out"=w905:errorcluster, "EotDetected"=→"EotLeftDetected3":bool, "axis"=w907:u8, "deviceHandle"=w906:i32)  [unwired: 5 in]
                        n398 = call "AMC_getStatusEotFwd.vi"("error in"=w905, "axis"=w907, "deviceHandle"=w906) -> ("error out"=w894:errorcluster, "EotDetected"=→"EotrightDetected3":bool, "axis"=w895:u8, "deviceHandle"=w896:i32)  [unwired: 5 in]
                        n399 = call "AMC_getStatusTargetRange.vi"("error in"=w894, "axis"=w895, "deviceHandle"=w896) -> ("error out"=w893:errorcluster, "in target range"=→"in target range3":bool)  [unwired: 5 in, 2 out]
                      }
                    }
                    n400 = Unbundle(w728) -> ("code"=w727:i32, "source"=w729:string)  [unwired: 1 out]
                    n401 = Not Equal To 0?(x=w727) -> (x != 0?=w726:bool)
                    n402 = case shown="True" w726 {
                      selector: w726 -> [_ w733]
                      tunnel: w729 -> [_ w734]
                      frame False {
                      }
                      frame True {
                        "Error Message 3" <- w734
                        "Error 3" <- w733
                      }
                    }
                  }
                }
              }
              frame "Interface" {
                n403 = stacked-sequence {
                  tunnel: w919 -> [w926 w1050 w1173]
                  frame #0 {
                    w925 = u8 0 items=["1", "2", "3"] ("axis in")
                    n404 = event shown="[4] \"Change per pulse 1\": Value Change" {
                      selector: _ -> [_ _ _ _ _ _ _ _ _ _ _]
                      dyn-events: _ -> [_ _ _ _ _ _ _ _ _ _ _]
                      timeout: 1 -> [_ _ _ _ _ _ _ _ _ _ _]
                      tunnel: w926 -> [w938 w961 w971 w982 w992 w1002 w1010 w1021 w1032 w1041 _]
                      tunnel: w925 -> [w936 w960 w970 w981 w991 w1001 w1009 w1022 w1031 w1038 _]
                      tunnel: [_ w948 w963 w972 w987 w995 w1004 w1015 w1027 w1034 _] -> w922
                      event Timeout {
                        n405 = event-data() -> ()  [unwired: 1 in, 1 out]
                        n406 = call "AMC_controlRealtimeInputMode.vi"("set"=FALSE, "axis"=w936, "deviceHandle"=w938) -> ("mode out"=w930:i32, "axis"=w935:u8, "deviceHandle"=w937:i32)  [unwired: 5 in, 1 out]
                        n407 = local write "Mode Input 1"(w930) -> ()
                        n408 = Equal?(x=w930, y=15) -> (x = y?=w933:bool)
                        n409 = call "AMC_controlRealtimeInputLoopMode.vi"("set"=FALSE, "axis"=w935, "deviceHandle"=w937) -> ("mode out"=w929:i32)  [unwired: 5 in, 3 out]
                        n410 = local write "Loop Mode 1"(w929) -> ()
                        n411 = Equal?(x=w929, y=0) -> (x = y?=w931:bool)
                        n412 = case shown="False" w933 {
                          tunnel: w931 -> [w941 _]
                          frame False {
                            n413 = case shown="True" w941 {
                              frame False {
                                w942 = T1."Enabled" ("Disabled")
                                n414 = property on="RT in move 1" class="Bool (strict)"("DisabledEnum"=w942) -> ()  [unwired: 2 in, 2 out]
                                n415 = property on="RT in move Signal 1" class="Bool (strict)"("DisabledEnum"=w942) -> ()  [unwired: 2 in, 2 out]
                                n416 = property on="Loop Mode 1" class="Ring (strict)"("DisabledEnum"=w942) -> ()  [unwired: 2 in, 2 out]
                                n417 = property on="Steps per pulse 1" class="DigNum (strict)"("DisabledEnum"=T1."Disabled and Grayed Out" ("Disabled")) -> ()  [unwired: 2 in, 2 out]
                                n418 = property on="Change per pulse 1" class="DigNum (strict)"("DisabledEnum"=w942) -> ()  [unwired: 2 in, 2 out]
                              }
                              frame True {
                                w945 = T1."Enabled" ("Disabled")
                                w944 = T1."Disabled and Grayed Out" ("Disabled")
                                n419 = property on="RT in move 1" class="Bool (strict)"("DisabledEnum"=w944) -> ()  [unwired: 2 in, 2 out]
                                n420 = property on="RT in move Signal 1" class="Bool (strict)"("DisabledEnum"=w944) -> ()  [unwired: 2 in, 2 out]
                                n421 = property on="Loop Mode 1" class="Ring (strict)"("DisabledEnum"=w945) -> ()  [unwired: 2 in, 2 out]
                                n422 = property on="Steps per pulse 1" class="DigNum (strict)"("DisabledEnum"=w945) -> ()  [unwired: 2 in, 2 out]
                                n423 = property on="Change per pulse 1" class="DigNum (strict)"("DisabledEnum"=w944) -> ()  [unwired: 2 in, 2 out]
                              }
                            }
                          }
                          frame True {
                            w946 = T1."Disabled and Grayed Out" ("Disabled")
                            n424 = property on="RT in move 1" class="Bool (strict)"("DisabledEnum"=w946) -> ()  [unwired: 2 in, 2 out]
                            n425 = property on="RT in move Signal 1" class="Bool (strict)"("DisabledEnum"=w946) -> ()  [unwired: 2 in, 2 out]
                            n426 = property on="Loop Mode 1" class="Ring (strict)"("DisabledEnum"=w946) -> ()  [unwired: 2 in, 2 out]
                            n427 = property on="Steps per pulse 1" class="DigNum (strict)"("DisabledEnum"=w946) -> ()  [unwired: 2 in, 2 out]
                            n428 = property on="Change per pulse 1" class="DigNum (strict)"("DisabledEnum"=w946) -> ()  [unwired: 2 in, 2 out]
                          }
                        }
                      }
                      event "Mode Input 1": Value Change {
                        n429 = event-data() -> ()  [unwired: 1 in, 1 out]
                        n430 = call "AMC_controlRealtimeInputMode.vi"("set"=TRUE, "mode in"="Mode Input 1", "axis"=w960, "deviceHandle"=w961) -> ("error out"=w955:errorcluster, "axis"=w956:u8, "deviceHandle"=w957:i32)  [unwired: 4 in, 1 out]
                        n431 = call "AMC_controlRealtimeInputMode.vi"("set"=FALSE, "error in"=w955, "axis"=w956, "deviceHandle"=w957) -> ("error out"=w949:errorcluster, "mode out"=w953:i32, "axis"=w950:u8, "deviceHandle"=w951:i32)  [unwired: 4 in]
                        n432 = local write "Mode Input 1"(w953) -> ()
                        n433 = call "AMC_controlRealtimeInputLoopMode.vi"("set"=FALSE, "error in"=w949, "axis"=w950, "deviceHandle"=w951) -> ("error out"=w948:errorcluster, "mode out"=w947:i32)  [unwired: 4 in, 2 out]
                        n434 = local write "Loop Mode 1"(w947) -> ()
                      }
                      event "Loop Mode 1": Value Change {
                        n435 = event-data() -> ()  [unwired: 1 in, 1 out]
                        n436 = call "AMC_controlRealtimeInputLoopMode.vi"("set"=TRUE, "mode in"="Loop Mode 1", "axis"=w970, "deviceHandle"=w971) -> ("error out"=w964:errorcluster, "axis"=w968:u8, "deviceHandle"=w969:i32)  [unwired: 4 in, 1 out]
                        n437 = call "AMC_controlRealtimeInputLoopMode.vi"("set"=FALSE, "error in"=w964, "axis"=w968, "deviceHandle"=w969) -> ("error out"=w963:errorcluster, "mode out"=w962:i32)  [unwired: 4 in, 2 out]
                        n438 = local write "Loop Mode 1"(w962) -> ()
                      }
                      event "Steps per pulse 1": Value Change {
                        n439 = event-data() -> ()  [unwired: 1 in, 1 out]
                        n440 = call "AMC_controlRealtimeInputStepsPerPulse.vi"("set"=TRUE, "steps in"="Steps per pulse 1", "axis"=w981, "deviceHandle"=w982) -> ("error out"=w973:errorcluster, "axis"=w979:u8, "deviceHandle"=w980:i32)  [unwired: 4 in, 1 out]
                        n441 = call "AMC_controlRealtimeInputStepsPerPulse.vi"("set"=FALSE, "axis"=w979, "deviceHandle"=w980) -> ("error out"=w974:errorcluster, "steps out"=w975:i32)  [unwired: 5 in, 2 out]
                        n442 = local write "Steps per pulse 1"(w975) -> ()
                        n443 = Merge Errors(w974, w973) -> (w972:errorcluster)
                      }
                      event "Change per pulse 1": Value Change {
                        n444 = event-data() -> ()  [unwired: 1 in, 1 out]
                        n445 = call "AMC_controlRealtimeInputChangePerPulse.vi"("set"=TRUE, "change in"="Change per pulse 1", "axis"=w991, "deviceHandle"=w992) -> ("error out"=w988:errorcluster, "axis"=w989:u8, "deviceHandle"=w990:i32)  [unwired: 4 in, 1 out]
                        n446 = call "AMC_controlRealtimeInputChangePerPulse.vi"("set"=FALSE, "error in"=w988, "axis"=w989, "deviceHandle"=w990) -> ("error out"=w987:errorcluster, "change out"=w983:i32)  [unwired: 4 in, 2 out]
                        n447 = local write "Change per pulse 1"(w983) -> ()
                      }
                      event "RT in move 1": Value Change {
                        n448 = event-data() -> ()  [unwired: 1 in, 1 out]
                        n449 = call "AMC_controlRealtimeInputMove.vi"("set"=TRUE, "enable in"="RT in move 1", "axis"=w1001, "deviceHandle"=w1002) -> ("error out"=w996:errorcluster, "axis"=w997:u8, "deviceHandle"=w998:i32)  [unwired: 4 in, 1 out]
                        n450 = call "AMC_controlRealtimeInputMove.vi"("set"=FALSE, "error in"=w996, "axis"=w997, "deviceHandle"=w998) -> ("error out"=w995:errorcluster, "enable out"=→"RT in move Signal 1":bool)  [unwired: 4 in, 2 out]
                      }
                      event "AquadB in res 1": Value Change {
                        n451 = event-data() -> ()  [unwired: 1 in, 1 out]
                        n452 = call "AMC_controlAQuadBInResolution.vi"("set"=TRUE, "resolution in"="AquadB in res 1", "axis"=w1009, "deviceHandle"=w1010) -> ("error out"=w1006:errorcluster, "axis"=w1007:u8, "deviceHandle"=w1008:i32)  [unwired: 4 in, 1 out]
                        n453 = call "AMC_controlAQuadBInResolution.vi"("set"=FALSE, "error in"=w1006, "axis"=w1007, "deviceHandle"=w1008) -> ("error out"=w1004:errorcluster, "resolution out"=w1003:i32)  [unwired: 4 in, 2 out]
                        n454 = local write "AquadB in res 1"(w1003) -> ()
                      }
                      event "AquadB out 1": Value Change {
                        n455 = event-data() -> ()  [unwired: 1 in, 1 out]
                        n456 = call "AMC_controlAQuadBOut.vi"("set"=TRUE, "enable in"="AquadB out 1", "axis"=w1022, "deviceHandle"=w1021) -> ("error out"=w1016:errorcluster, "axis"=w1017:u8, "deviceHandle"=w1018:i32)  [unwired: 4 in, 1 out]
                        n457 = call "AMC_controlAQuadBOut.vi"("set"=FALSE, "error in"=w1016, "axis"=w1017, "deviceHandle"=w1018) -> ("error out"=w1015:errorcluster, "enable out"=w1013:bool)  [unwired: 4 in, 2 out]
                        n458 = local write "AquadB out 1"(w1013) -> ()
                      }
                      event "AqaudB clock 1": Value Change {
                        (unwired) TRUE ("set")
                        n459 = event-data() -> ()  [unwired: 1 in, 1 out]
                        n460 = call "AMC_controlAQuadBOutClock.vi"("set"=TRUE, "clock in"="AqaudB clock 1", "axis"=w1031, "deviceHandle"=w1032) -> ("error out"=w1028:errorcluster, "axis"=w1024:u8, "deviceHandle"=w1025:i32)  [unwired: 4 in, 1 out]
                        n461 = call "AMC_controlAQuadBOutClock.vi"("set"=FALSE, "error in"=w1028, "axis"=w1024, "deviceHandle"=w1025) -> ("error out"=w1027:errorcluster, "clock out"=w1026:i32)  [unwired: 4 in, 2 out]
                        n462 = local write "AqaudB clock 1"(w1026) -> ()
                      }
                      event "AquadB Resolution 1": Value Change {
                        n463 = event-data() -> ()  [unwired: 1 in, 1 out]
                        n464 = call "AMC_controlAQuadBOutResolution.vi"("set"=TRUE, "resolution in"="AquadB Resolution 1", "axis"=w1038, "deviceHandle"=w1041) -> ("axis"=w1035:u8, "deviceHandle"=w1036:i32)  [unwired: 4 in, 2 out]
                        n465 = call "AMC_controlAQuadBOutResolution.vi"("set"=FALSE, "axis"=w1035, "deviceHandle"=w1036) -> ("error out"=w1034:errorcluster, "resolution out"=w1033:i32)  [unwired: 5 in, 2 out]
                        n466 = local write "AquadB Resolution 1"(w1033) -> ()
                      }
                      event "Reset Error 4": Value Change {
                        n467 = event-data() -> ()  [unwired: 1 in, 1 out]
                        n468 = local write "Error Message 4"("" ("Error Message")) -> ()
                        n469 = local write "Error 4"(FALSE ("Error 4")) -> ()
                      }
                    }
                    n470 = Unbundle(w922) -> ("code"=w920:i32, "source"=w921:string)  [unwired: 1 out]
                    n471 = Not Equal To 0?(x=w920) -> (x != 0?=w923:bool)
                    n472 = case shown="True" w923 {
                      selector: w923 -> [_ w927]
                      tunnel: w921 -> [_ w928]
                      frame False {
                      }
                      frame True {
                        "Error Message 4" <- w928
                        "Error 4" <- w927
                      }
                    }
                  }
                  frame #1 {
                    w1049 = u8 1 items=["1", "2", "3"] ("axis in")
                    n473 = event shown="[4] \"Change per pulse 2\": Value Change" {
                      selector: _ -> [_ _ _ _ _ _ _ _ _ _ _]
                      dyn-events: _ -> [_ _ _ _ _ _ _ _ _ _ _]
                      timeout: 1 -> [_ _ _ _ _ _ _ _ _ _ _]
                      tunnel: w1050 -> [w1056 w1081 w1090 w1101 w1110 w1120 w1133 w1144 w1154 w1164 _]
                      tunnel: w1049 -> [w1055 w1079 w1087 w1098 w1109 w1118 w1132 w1145 w1153 w1163 _]
                      tunnel: [_ w1072 w1089 w1099 w1108 w1116 w1127 w1138 w1147 w1157 _] -> w1044
                      event Timeout {
                        n474 = event-data() -> ()  [unwired: 1 in, 1 out]
                        n475 = call "AMC_controlRealtimeInputMode.vi"("set"=FALSE, "axis"=w1055, "deviceHandle"=w1056) -> ("mode out"=w1054:i32, "axis"=w1061:u8, "deviceHandle"=w1062:i32)  [unwired: 5 in, 1 out]
                        n476 = local write "Mode Input 2"(w1054) -> ()
                        n477 = Equal?(x=w1054, y=15) -> (x = y?=w1059:bool)
                        n478 = call "AMC_controlRealtimeInputLoopMode.vi"("set"=FALSE, "axis"=w1061, "deviceHandle"=w1062) -> ("mode out"=w1053:i32)  [unwired: 5 in, 3 out]
                        n479 = local write "Loop Mode 2"(w1053) -> ()
                        n480 = Equal?(x=w1053, y=0) -> (x = y?=w1057:bool)
                        n481 = case shown="False" w1059 {
                          tunnel: w1057 -> [w1065 _]
                          frame False {
                            n482 = case shown="False" w1065 {
                              frame False {
                                w1066 = T1."Enabled" ("Disabled")
                                n483 = property on="RT in move 2" class="Bool (strict)"("DisabledEnum"=w1066) -> ()  [unwired: 2 in, 2 out]
                                n484 = property on="RT in move Signal 2" class="Bool (strict)"("DisabledEnum"=w1066) -> ()  [unwired: 2 in, 2 out]
                                n485 = property on="Loop Mode 2" class="Ring (strict)"("DisabledEnum"=w1066) -> ()  [unwired: 2 in, 2 out]
                                n486 = property on="Steps per pulse 2" class="DigNum (strict)"("DisabledEnum"=T1."Disabled and Grayed Out" ("Disabled")) -> ()  [unwired: 2 in, 2 out]
                                n487 = property on="Change per pulse 2" class="DigNum (strict)"("DisabledEnum"=w1066) -> ()  [unwired: 2 in, 2 out]
                              }
                              frame True {
                                w1069 = T1."Enabled" ("Disabled")
                                w1068 = T1."Disabled and Grayed Out" ("Disabled")
                                n488 = property on="RT in move 2" class="Bool (strict)"("DisabledEnum"=w1068) -> ()  [unwired: 2 in, 2 out]
                                n489 = property on="RT in move Signal 2" class="Bool (strict)"("DisabledEnum"=w1068) -> ()  [unwired: 2 in, 2 out]
                                n490 = property on="Loop Mode 2" class="Ring (strict)"("DisabledEnum"=w1069) -> ()  [unwired: 2 in, 2 out]
                                n491 = property on="Steps per pulse 2" class="DigNum (strict)"("DisabledEnum"=w1069) -> ()  [unwired: 2 in, 2 out]
                                n492 = property on="Change per pulse 2" class="DigNum (strict)"("DisabledEnum"=w1068) -> ()  [unwired: 2 in, 2 out]
                              }
                            }
                          }
                          frame True {
                            w1070 = T1."Disabled and Grayed Out" ("Disabled")
                            n493 = property on="RT in move 2" class="Bool (strict)"("DisabledEnum"=w1070) -> ()  [unwired: 2 in, 2 out]
                            n494 = property on="RT in move Signal 2" class="Bool (strict)"("DisabledEnum"=w1070) -> ()  [unwired: 2 in, 2 out]
                            n495 = property on="Loop Mode 2" class="Ring (strict)"("DisabledEnum"=w1070) -> ()  [unwired: 2 in, 2 out]
                            n496 = property on="Steps per pulse 2" class="DigNum (strict)"("DisabledEnum"=w1070) -> ()  [unwired: 2 in, 2 out]
                            n497 = property on="Change per pulse 2" class="DigNum (strict)"("DisabledEnum"=w1070) -> ()  [unwired: 2 in, 2 out]
                          }
                        }
                      }
                      event "Mode Input 2": Value Change {
                        n498 = event-data() -> ()  [unwired: 1 in, 1 out]
                        n499 = call "AMC_controlRealtimeInputMode.vi"("set"=TRUE, "mode in"="Mode Input 2", "axis"=w1079, "deviceHandle"=w1081) -> ("error out"=w1077:errorcluster, "axis"=w1083:u8, "deviceHandle"=w1084:i32)  [unwired: 4 in, 1 out]
                        n500 = call "AMC_controlRealtimeInputMode.vi"("set"=FALSE, "error in"=w1077, "axis"=w1083, "deviceHandle"=w1084) -> ("error out"=w1073:errorcluster, "mode out"=w1078:i32, "axis"=w1074:u8, "deviceHandle"=w1075:i32)  [unwired: 4 in]
                        n501 = local write "Mode Input 2"(w1078) -> ()
                        n502 = call "AMC_controlRealtimeInputLoopMode.vi"("set"=FALSE, "error in"=w1073, "axis"=w1074, "deviceHandle"=w1075) -> ("error out"=w1072:errorcluster, "mode out"=w1071:i32)  [unwired: 4 in, 2 out]
                        n503 = local write "Loop Mode 2"(w1071) -> ()
                      }
                      event "Loop Mode 2": Value Change {
                        n504 = event-data() -> ()  [unwired: 1 in, 1 out]
                        n505 = call "AMC_controlRealtimeInputLoopMode.vi"("set"=TRUE, "mode in"="Loop Mode 2", "axis"=w1087, "deviceHandle"=w1090) -> ("error out"=w1091:errorcluster, "axis"=w1094:u8, "deviceHandle"=w1095:i32)  [unwired: 4 in, 1 out]
                        n506 = call "AMC_controlRealtimeInputLoopMode.vi"("set"=FALSE, "error in"=w1091, "axis"=w1094, "deviceHandle"=w1095) -> ("error out"=w1089:errorcluster, "mode out"=w1086:i32)  [unwired: 4 in, 2 out]
                        n507 = local write "Loop Mode 2"(w1086) -> ()
                      }
                      event "Steps per pulse 2": Value Change {
                        n508 = event-data() -> ()  [unwired: 1 in, 1 out]
                        n509 = call "AMC_controlRealtimeInputStepsPerPulse.vi"("set"=TRUE, "steps in"="Steps per pulse 2", "axis"=w1098, "deviceHandle"=w1101) -> ("error out"=w1100:errorcluster, "axis"=w1104:u8, "deviceHandle"=w1105:i32)  [unwired: 4 in, 1 out]
                        n510 = call "AMC_controlRealtimeInputStepsPerPulse.vi"("set"=FALSE, "error in"=w1100, "axis"=w1104, "deviceHandle"=w1105) -> ("error out"=w1099:errorcluster, "steps out"=w1096:i32)  [unwired: 4 in, 2 out]
                        n511 = local write "Steps per pulse 2"(w1096) -> ()
                      }
                      event "Change per pulse 2": Value Change {
                        n512 = event-data() -> ()  [unwired: 1 in, 1 out]
                        n513 = call "AMC_controlRealtimeInputChangePerPulse.vi"("set"=TRUE, "change in"="Change per pulse 2", "axis"=w1109, "deviceHandle"=w1110) -> ("error out"=w1113:errorcluster, "axis"=w1114:u8, "deviceHandle"=w1115:i32)  [unwired: 4 in, 1 out]
                        n514 = call "AMC_controlRealtimeInputChangePerPulse.vi"("set"=FALSE, "error in"=w1113, "axis"=w1114, "deviceHandle"=w1115) -> ("error out"=w1108:errorcluster, "change out"=w1106:i32)  [unwired: 4 in, 2 out]
                        n515 = local write "Change per pulse 2"(w1106) -> ()
                      }
                      event "RT in move 2": Value Change {
                        n516 = event-data() -> ()  [unwired: 1 in, 1 out]
                        n517 = call "AMC_controlRealtimeInputMove.vi"("set"=TRUE, "enable in"="RT in move 2", "axis"=w1118, "deviceHandle"=w1120) -> ("error out"=w1122:errorcluster, "axis"=w1123:u8, "deviceHandle"=w1124:i32)  [unwired: 4 in, 1 out]
                        n518 = call "AMC_controlRealtimeInputMove.vi"("set"=FALSE, "error in"=w1122, "axis"=w1123, "deviceHandle"=w1124) -> ("error out"=w1116:errorcluster, "enable out"=→"RT in move Signal 2":bool)  [unwired: 4 in, 2 out]
                      }
                      event "AquadB in res 2": Value Change {
                        n519 = event-data() -> ()  [unwired: 1 in, 1 out]
                        n520 = call "AMC_controlAQuadBInResolution.vi"("set"=TRUE, "resolution in"="AquadB in res 2", "axis"=w1132, "deviceHandle"=w1133) -> ("error out"=w1129:errorcluster, "axis"=w1130:u8, "deviceHandle"=w1131:i32)  [unwired: 4 in, 1 out]
                        n521 = call "AMC_controlAQuadBInResolution.vi"("set"=FALSE, "error in"=w1129, "axis"=w1130, "deviceHandle"=w1131) -> ("error out"=w1127:errorcluster, "resolution out"=w1126:i32)  [unwired: 4 in, 2 out]
                        n522 = local write "AquadB in res 2"(w1126) -> ()
                      }
                      event "AquadB out 2": Value Change {
                        n523 = event-data() -> ()  [unwired: 1 in, 1 out]
                        n524 = call "AMC_controlAQuadBOut.vi"("set"=TRUE, "enable in"="AquadB out 2", "axis"=w1145, "deviceHandle"=w1144) -> ("error out"=w1139:errorcluster, "axis"=w1140:u8, "deviceHandle"=w1141:i32)  [unwired: 4 in, 1 out]
                        n525 = call "AMC_controlAQuadBOut.vi"("set"=FALSE, "error in"=w1139, "axis"=w1140, "deviceHandle"=w1141) -> ("error out"=w1138:errorcluster, "enable out"=w1136:bool)  [unwired: 4 in, 2 out]
                        n526 = local write "AquadB out 2"(w1136) -> ()
                      }
                      event "AqaudB clock 2": Value Change {
                        n527 = event-data() -> ()  [unwired: 1 in, 1 out]
                        n528 = call "AMC_controlAQuadBOutClock.vi"("set"=TRUE, "clock in"="AqaudB clock 2", "axis"=w1153, "deviceHandle"=w1154) -> ("error out"=w1148:errorcluster, "axis"=w1149:u8, "deviceHandle"=w1150:i32)  [unwired: 4 in, 1 out]
                        n529 = call "AMC_controlAQuadBOutClock.vi"("set"=FALSE, "error in"=w1148, "axis"=w1149, "deviceHandle"=w1150) -> ("error out"=w1147:errorcluster, "clock out"=w1146:i32)  [unwired: 4 in, 2 out]
                        n530 = local write "AqaudB clock 2"(w1146) -> ()
                      }
                      event "AquadB Resolution 2": Value Change {
                        n531 = event-data() -> ()  [unwired: 1 in, 1 out]
                        n532 = call "AMC_controlAQuadBOutResolution.vi"("set"=TRUE, "resolution in"="AquadB Resolution 2", "axis"=w1163, "deviceHandle"=w1164) -> ("error out"=w1158:errorcluster, "axis"=w1159:u8, "deviceHandle"=w1160:i32)  [unwired: 4 in, 1 out]
                        n533 = call "AMC_controlAQuadBOutResolution.vi"("set"=FALSE, "error in"=w1158, "axis"=w1159, "deviceHandle"=w1160) -> ("error out"=w1157:errorcluster, "resolution out"=w1156:i32)  [unwired: 4 in, 2 out]
                        n534 = local write "AquadB Resolution 2"(w1156) -> ()
                      }
                      event "Reset Error 5": Value Change {
                        n535 = event-data() -> ()  [unwired: 1 in, 1 out]
                        n536 = local write "Error 5"(FALSE ("Error 5")) -> ()
                        n537 = local write "Error Message 5"("" ("Error Message")) -> ()
                      }
                    }
                    n538 = Unbundle(w1044) -> ("code"=w1046:i32, "source"=w1045:string)  [unwired: 1 out]
                    n539 = Not Equal To 0?(x=w1046) -> (x != 0?=w1047:bool)
                    n540 = case shown="True" w1047 {
                      selector: w1047 -> [_ w1051]
                      tunnel: w1045 -> [_ w1052]
                      frame False {
                      }
                      frame True {
                        "Error Message 5" <- w1052
                        "Error 5" <- w1051
                      }
                    }
                  }
                  frame #2 {
                    w1172 = u8 2 items=["1", "2", "3"] ("axis in")
                    n541 = event shown="[4] \"Change per pulse 3\": Value Change" {
                      selector: _ -> [_ _ _ _ _ _ _ _ _ _ _ _]
                      dyn-events: _ -> [_ _ _ _ _ _ _ _ _ _ _ _]
                      timeout: 1 -> [_ _ _ _ _ _ _ _ _ _ _ _]
                      tunnel: w1173 -> [w1180 w1204 w1214 w1224 w1234 w1244 w1257 w1266 w1277 w1286 w1296 _]
                      tunnel: w1172 -> [w1179 w1203 w1212 w1223 w1232 w1243 w1256 _ w1278 w1285 w1295 _]
                      tunnel: [_ w1196 w1213 w1221 w1233 w1242 w1252 w1262 w1271 w1280 w1290 _] -> w1168
                      event Timeout {
                        n542 = event-data() -> ()  [unwired: 1 in, 1 out]
                        n543 = call "AMC_controlRealtimeInputMode.vi"("set"=FALSE, "axis"=w1179, "deviceHandle"=w1180) -> ("mode out"=w1178:i32, "axis"=w1185:u8, "deviceHandle"=w1186:i32)  [unwired: 5 in, 1 out]
                        n544 = local write "Mode Input 3"(w1178) -> ()
                        n545 = Equal?(x=w1178, y=15) -> (x = y?=w1183:bool)
                        n546 = call "AMC_controlRealtimeInputLoopMode.vi"("set"=FALSE, "axis"=w1185, "deviceHandle"=w1186) -> ("mode out"=w1177:i32)  [unwired: 5 in, 3 out]
                        n547 = local write "Loop Mode 3"(w1177) -> ()
                        n548 = Equal?(x=w1177, y=0) -> (x = y?=w1181:bool)
                        n549 = case shown="False" w1183 {
                          tunnel: w1181 -> [w1189 _]
                          frame False {
                            n550 = case shown="True" w1189 {
                              frame False {
                                w1190 = T1."Enabled" ("Disabled")
                                n551 = property on="RT in move 3" class="Bool (strict)"("DisabledEnum"=w1190) -> ()  [unwired: 2 in, 2 out]
                                n552 = property on="RT in move Signal 3" class="Bool (strict)"("DisabledEnum"=w1190) -> ()  [unwired: 2 in, 2 out]
                                n553 = property on="Loop Mode 3" class="Ring (strict)"("DisabledEnum"=w1190) -> ()  [unwired: 2 in, 2 out]
                                n554 = property on="Steps per pulse 3" class="DigNum (strict)"("DisabledEnum"=T1."Disabled and Grayed Out" ("Disabled")) -> ()  [unwired: 2 in, 2 out]
                                n555 = property on="Change per pulse 3" class="DigNum (strict)"("DisabledEnum"=w1190) -> ()  [unwired: 2 in, 2 out]
                              }
                              frame True {
                                w1193 = T1."Enabled" ("Disabled")
                                w1192 = T1."Disabled and Grayed Out" ("Disabled")
                                n556 = property on="RT in move 3" class="Bool (strict)"("DisabledEnum"=w1192) -> ()  [unwired: 2 in, 2 out]
                                n557 = property on="RT in move Signal 3" class="Bool (strict)"("DisabledEnum"=w1192) -> ()  [unwired: 2 in, 2 out]
                                n558 = property on="Loop Mode 3" class="Ring (strict)"("DisabledEnum"=w1193) -> ()  [unwired: 2 in, 2 out]
                                n559 = property on="Steps per pulse 3" class="DigNum (strict)"("DisabledEnum"=w1193) -> ()  [unwired: 2 in, 2 out]
                                n560 = property on="Change per pulse 3" class="DigNum (strict)"("DisabledEnum"=w1192) -> ()  [unwired: 2 in, 2 out]
                              }
                            }
                          }
                          frame True {
                            w1194 = T1."Disabled and Grayed Out" ("Disabled")
                            n561 = property on="RT in move 3" class="Bool (strict)"("DisabledEnum"=w1194) -> ()  [unwired: 2 in, 2 out]
                            n562 = property on="RT in move Signal 3" class="Bool (strict)"("DisabledEnum"=w1194) -> ()  [unwired: 2 in, 2 out]
                            n563 = property on="Loop Mode 3" class="Ring (strict)"("DisabledEnum"=w1194) -> ()  [unwired: 2 in, 2 out]
                            n564 = property on="Steps per pulse 3" class="DigNum (strict)"("DisabledEnum"=w1194) -> ()  [unwired: 2 in, 2 out]
                            n565 = property on="Change per pulse 3" class="DigNum (strict)"("DisabledEnum"=w1194) -> ()  [unwired: 2 in, 2 out]
                          }
                        }
                      }
                      event "Mode Input 3": Value Change {
                        n566 = event-data() -> ()  [unwired: 1 in, 1 out]
                        n567 = call "AMC_controlRealtimeInputMode.vi"("set"=TRUE, "mode in"="Mode Input 3", "axis"=w1203, "deviceHandle"=w1204) -> ("error out"=w1206:errorcluster, "axis"=w1207:u8, "deviceHandle"=w1208:i32)  [unwired: 4 in, 1 out]
                        n568 = call "AMC_controlRealtimeInputMode.vi"("set"=FALSE, "error in"=w1206, "axis"=w1207, "deviceHandle"=w1208) -> ("error out"=w1197:errorcluster, "mode out"=w1201:i32, "axis"=w1198:u8, "deviceHandle"=w1199:i32)  [unwired: 4 in]
                        n569 = local write "Mode Input 3"(w1201) -> ()
                        n570 = call "AMC_controlRealtimeInputLoopMode.vi"("set"=FALSE, "error in"=w1197, "axis"=w1198, "deviceHandle"=w1199) -> ("error out"=w1196:errorcluster, "mode out"=w1195:i32)  [unwired: 4 in, 2 out]
                        n571 = local write "Loop Mode 3"(w1195) -> ()
                      }
                      event "Loop Mode 3": Value Change {
                        n572 = event-data() -> ()  [unwired: 1 in, 1 out]
                        n573 = call "AMC_controlRealtimeInputLoopMode.vi"("set"=TRUE, "mode in"="Loop Mode 3", "axis"=w1212, "deviceHandle"=w1214) -> ("error out"=w1219:errorcluster, "axis"=w1216:u8, "deviceHandle"=w1215:i32)  [unwired: 4 in, 1 out]
                        n574 = call "AMC_controlRealtimeInputLoopMode.vi"("set"=FALSE, "error in"=w1219, "axis"=w1216, "deviceHandle"=w1215) -> ("error out"=w1213:errorcluster, "mode out"=w1210:i32)  [unwired: 4 in, 2 out]
                        n575 = local write "Loop Mode 3"(w1210) -> ()
                      }
                      event "Steps per pulse 3": Value Change {
                        n576 = event-data() -> ()  [unwired: 1 in, 1 out]
                        n577 = call "AMC_controlRealtimeInputStepsPerPulse.vi"("set"=TRUE, "steps in"="Steps per pulse 3", "axis"=w1223, "deviceHandle"=w1224) -> ("error out"=w1229:errorcluster, "axis"=w1226:u8, "deviceHandle"=w1225:i32)  [unwired: 4 in, 1 out]
                        n578 = call "AMC_controlRealtimeInputStepsPerPulse.vi"("set"=FALSE, "error in"=w1229, "axis"=w1226, "deviceHandle"=w1225) -> ("error out"=w1221:errorcluster, "steps out"=w1220:i32)  [unwired: 4 in, 2 out]
                        n579 = local write "Steps per pulse 3"(w1220) -> ()
                      }
                      event "Change per pulse 3": Value Change {
                        n580 = event-data() -> ()  [unwired: 1 in, 1 out]
                        n581 = call "AMC_controlRealtimeInputChangePerPulse.vi"("set"=TRUE, "change in"="Change per pulse 3", "axis"=w1232, "deviceHandle"=w1234) -> ("error out"=w1237:errorcluster, "axis"=w1236:u8, "deviceHandle"=w1235:i32)  [unwired: 4 in, 1 out]
                        n582 = call "AMC_controlRealtimeInputChangePerPulse.vi"("set"=FALSE, "error in"=w1237, "axis"=w1236, "deviceHandle"=w1235) -> ("error out"=w1233:errorcluster, "change out"=w1230:i32)  [unwired: 4 in, 2 out]
                        n583 = local write "Change per pulse 3"(w1230) -> ()
                      }
                      event "RT in move 3": Value Change {
                        n584 = event-data() -> ()  [unwired: 1 in, 1 out]
                        n585 = call "AMC_controlRealtimeInputMove.vi"("set"=TRUE, "enable in"="RT in move 3", "axis"=w1243, "deviceHandle"=w1244) -> ("error out"=w1248:errorcluster, "axis"=w1247:u8, "deviceHandle"=w1246:i32)  [unwired: 4 in, 1 out]
                        n586 = call "AMC_controlRealtimeInputMove.vi"("set"=FALSE, "error in"=w1248, "axis"=w1247, "deviceHandle"=w1246) -> ("error out"=w1242:errorcluster, "enable out"=→"RT in move Signal 3":bool)  [unwired: 4 in, 2 out]
                      }
                      event "AquadB in res 3": Value Change {
                        n587 = event-data() -> ()  [unwired: 1 in, 1 out]
                        n588 = call "AMC_controlAQuadBInResolution.vi"("set"=TRUE, "resolution in"="AquadB in res 3", "axis"=w1256, "deviceHandle"=w1257) -> ("error out"=w1253:errorcluster, "axis"=w1254:u8, "deviceHandle"=w1255:i32)  [unwired: 4 in, 1 out]
                        n589 = call "AMC_controlAQuadBInResolution.vi"("set"=FALSE, "error in"=w1253, "axis"=w1254, "deviceHandle"=w1255) -> ("error out"=w1252:errorcluster, "resolution out"=w1250:i32)  [unwired: 4 in, 2 out]
                        n590 = local write "AquadB in res 3"(w1250) -> ()
                      }
                      event "Output Mode": Value Change {
                        n591 = event-data() -> ()  [unwired: 1 in, 1 out]
                        n592 = call "AMC_controlRtOutSignalMode.vi"("deviceHandle"=w1266, "mode in"="Output Mode", "set"=TRUE) -> ("deviceHandle"=w1265:i32, "mode out"=w1264:i32, "error out"=w1263:errorcluster)  [unwired: 5 in]
                        n593 = call "AMC_controlRtOutSignalMode.vi"("deviceHandle"=w1265, "mode in"=w1264, "error in"=w1263, "set"=FALSE) -> ("mode out"=w1260:i32, "error out"=w1262:errorcluster)  [unwired: 4 in, 1 out]
                        n594 = local write "Output Mode"(w1260) -> ()
                      }
                      event "AquadB out 3": Value Change {
                        n595 = event-data() -> ()  [unwired: 1 in, 1 out]
                        n596 = call "AMC_controlAQuadBOut.vi"("set"=TRUE, "enable in"="AquadB out 3", "axis"=w1278, "deviceHandle"=w1277) -> ("error out"=w1272:errorcluster, "axis"=w1273:u8, "deviceHandle"=w1274:i32)  [unwired: 4 in, 1 out]
                        n597 = call "AMC_controlAQuadBOut.vi"("set"=FALSE, "error in"=w1272, "axis"=w1273, "deviceHandle"=w1274) -> ("error out"=w1271:errorcluster, "enable out"=w1269:bool)  [unwired: 4 in, 2 out]
                        n598 = local write "AquadB out 3"(w1269) -> ()
                      }
                      event "AqaudB clock 3": Value Change {
                        n599 = event-data() -> ()  [unwired: 1 in, 1 out]
                        n600 = call "AMC_controlAQuadBOutClock.vi"("set"=TRUE, "clock in"="AqaudB clock 3", "axis"=w1285, "deviceHandle"=w1286) -> ("error out"=w1281:errorcluster, "axis"=w1282:u8, "deviceHandle"=w1283:i32)  [unwired: 4 in, 1 out]
                        n601 = call "AMC_controlAQuadBOutClock.vi"("set"=FALSE, "error in"=w1281, "axis"=w1282, "deviceHandle"=w1283) -> ("error out"=w1280:errorcluster, "clock out"=w1279:i32)  [unwired: 4 in, 2 out]
                        n602 = local write "AqaudB clock 3"(w1279) -> ()
                      }
                      event "AquadB Resolution 3": Value Change {
                        n603 = event-data() -> ()  [unwired: 1 in, 1 out]
                        n604 = call "AMC_controlAQuadBOutResolution.vi"("set"=TRUE, "resolution in"="AquadB Resolution 3", "axis"=w1295, "deviceHandle"=w1296) -> ("error out"=w1293:errorcluster, "axis"=w1291:u8, "deviceHandle"=w1292:i32)  [unwired: 4 in, 1 out]
                        n605 = call "AMC_controlAQuadBOutResolution.vi"("set"=TRUE, "error in"=w1293, "axis"=w1291, "deviceHandle"=w1292) -> ("error out"=w1290:errorcluster, "resolution out"=w1289:i32)  [unwired: 4 in, 2 out]
                        n606 = local write "AquadB Resolution 3"(w1289) -> ()
                      }
                      event "Reset Error 6": Value Change {
                        n607 = event-data() -> ()  [unwired: 1 in, 1 out]
                        n608 = local write "Error 6"(FALSE ("Error 6")) -> ()
                        n609 = local write "Error Message 6"("" ("Error Message")) -> ()
                      }
                    }
                    n610 = Unbundle(w1168) -> ("code"=w1170:i32, "source"=w1171:string)  [unwired: 1 out]
                    n611 = Not Equal To 0?(x=w1170) -> (x != 0?=w1169:bool)
                    n612 = case shown="True" w1169 {
                      selector: w1169 -> [_ w1175]
                      tunnel: w1171 -> [_ w1176]
                      frame False {
                      }
                      frame True {
                        "Error Message 6" <- w1176
                        "Error 6" <- w1175
                      }
                    }
                  }
                }
              }
              frame "About" {
                n613 = event shown="[0] Timeout" {
                  selector: _ -> [_ _ _ _ _ _ _ _]
                  dyn-events: _ -> [_ _ _ _ _ _ _ _]
                  timeout: 1 -> [_ _ _ _ _ _ _ _]
                  tunnel: w1305 -> [w1315 w1317 w1320 w1323 w1325 w1328 w1330 _]
                  tunnel: [w1310 w1316 w1319 w1322 w1324 w1327 w1329 _] -> w1301
                  event Timeout {
                    n614 = event-data() -> ()  [unwired: 1 in, 1 out]
                    n615 = call "AMC_getLockStatus.vi"("deviceHandle"=w1315) -> ("error out"=w1311:errorcluster, "locked"=→"locked":bool, "authorized"=→"authorized":bool, "deviceHandle"=w1312:i32)  [unwired: 7 in]
                    n616 = call "AMC_getDeviceName.vi"("error in"=w1311, "deviceHandle"=w1312) -> ("error out"=w1310:errorcluster, "name"=→"Name":string)  [unwired: 7 in, 1 out]
                  }
                  event "name": Value Change {
                    n617 = event-data() -> ()  [unwired: 1 in, 1 out]
                    n618 = call "AMC_setDeviceName.vi"("name"="name", "deviceHandle"=w1317) -> ("error out"=w1316:errorcluster)  [unwired: 8 in, 1 out]
                  }
                  event "Lock password": Value Change {
                    n619 = event-data() -> ()  [unwired: 1 in, 1 out]
                    n620 = call "AMC_lock.vi"("password"="Lock password", "deviceHandle"=w1320) -> ("error out"=w1319:errorcluster)  [unwired: 8 in, 1 out]
                  }
                  event "Unlock": Value Change {
                    n621 = event-data() -> ()  [unwired: 1 in, 1 out]
                    n622 = call "AMC_unlock.vi"("deviceHandle"=w1323) -> ("error out"=w1322:errorcluster)  [unwired: 9 in, 1 out]
                  }
                  event "Access Password": Value Change {
                    n623 = event-data() -> ()  [unwired: 1 in, 1 out]
                    n624 = call "AMC_grantAccess.vi"("password"="Access Password", "deviceHandle"=w1325) -> ("error out"=w1324:errorcluster)  [unwired: 8 in, 1 out]
                  }
                  event "Reboot": Value Change {
                    n625 = event-data() -> ()  [unwired: 1 in, 1 out]
                    n626 = call "AMC_rebootSystem.vi"("deviceHandle"=w1328) -> ("error out"=w1327:errorcluster)  [unwired: 9 in, 1 out]
                  }
                  event "Factory Reset": Value Change {
                    n627 = event-data() -> ()  [unwired: 1 in, 1 out]
                    n628 = call "AMC_factoryReset.vi"("deviceHandle"=w1330) -> ("error out"=w1329:errorcluster)  [unwired: 9 in, 1 out]
                  }
                  event "Reset Error 7": Value Change {
                    n629 = event-data() -> ()  [unwired: 1 in, 1 out]
                    n630 = local write "Error 7"(FALSE ("Error 7")) -> ()
                    n631 = local write "Error Message 7"("" ("Error Message 9")) -> ()
                  }
                }
                n632 = Unbundle(w1301) -> ("code"=w1303:i32, "source"=w1304:string)  [unwired: 1 out]
                n633 = Not Equal To 0?(x=w1303) -> (x != 0?=w1302:bool)
                n634 = case shown="True" w1302 {
                  selector: w1302 -> [_ w1307]
                  tunnel: w1304 -> [_ w1308]
                  frame False {
                  }
                  frame True {
                    "Error Message 7" <- w1308
                    "Error 7" <- w1307
                  }
                }
              }
            }
          }
        }
        frame #2 {
          # "Disconnecting"
          n635 = call "AMC_close.vi"("deviceHandle"=w1333) -> ()  [unwired: 6 in, 1 out]
          n636 = local write "stop"(FALSE ("stop")) -> ()
        }
      }
    }
    frame True {
      # "No Devices Found"
      n637 = while {
        stop <- w1335 stop-if-true
        # "No Device Massage"
        n638 = One Button Dialog(message="No Devices Found", button name ("OK")="OK") -> (true=w1335:bool)
      }
    }
  }
